vi "Scope_5782_6channel_IQ_PID_Quench.vi"() -> ()   [LabVIEW 2018]
uses:
  FPGA/DataMode.ctl
  <vilib>/Analysis/4window.llb/windowTd.ctl
  Host/Scope/controls/power_spectrum_unit.ctl
  Host/Scope5782/Scope/controls/5782_trigger_type.ctl
  Host/Scope/controls/Data_calc_mode.ctl
  Host/Scope/controls/Data_display_mode.ctl
  Host/Scope/controls/Graph_references.ctl
  Host/Scope/controls/graph_controls.ctl
  Host/Scope/controls/Channel_select_2fpga.ctl
  FPGA/PID/PID control enabled type.ctl
  <vilib>/userdefined/High Color/nirio_resource_hc.ctl
  Host/Scope/controls/All FP controls.ctl
  Host/Scope/controls/Output scale.ctl
  Host/Scope/controls/host_transfer_speed.ctl
  FPGA/cavity model/Piezo setting.ctl
  Host/Scope/controls/w12 scale.ctl
  Host/Scope/controls/FFT buffer type.ctl
  Host/Communication/Driver/RemoteConnection/RemoteReferences.ctl
  Host/FpgaRef/FpgaRef5761/ClockSource_5761.ctl
  Host/INI files/Settings file IQ PID/SettingsFileIQpid.lvclass
  C:/PXIe/InProgress/source2/Host/INI files/Settings file base/SettingsFile.lvclass
  Host/Communication/Driver/RemoteConnection/RemoteConnection.lvclass
  Host/Scope/Scope5782_six_channel/Scope5782_six_channel.lvclass
  C:/PXIe/InProgress/source2/Host/Scope/ScopeBase/ScopeBase.lvclass
  FPGA/fpga_settings.ctl
  Host/INI files/Settings file base/Save event.ctl
  Host/Scope/Scope5782_six_channel/Scope5782_six_channel.lvclass/Scope5782_six_channel.ctl
  Host/Scope/controls/ScopeMode.ctl
  Host/FpgaRef/FpgaRef5761/FpgaRef5761.lvclass
  C:/PXIe/InProgress/source2/Host/FpgaRef/FpgaRefBase/FpgaRefBase.lvclass
  Host/FpgaRef/FpgaRef5782/FpgaRef5782.lvclass
  Host/Communication/global_stop.vi
  <vilib>/FPGAPlugInAG/PXIe-7975R/niLvFpga_Open_PXIe-7975R.vi
  <vilib>/rvi/interface/common/dynamic/niFpgaDynamicAddResources.vi
  <vilib>/Utility/error.llb/Error Cluster From Error Code.vi
  <vilib>/rvi/errors/niLvFpgaAdjustHostInterfaceError.vi
  Host/Communication/response.ctl
  Host/Communication/driver_status.ctl
  <vilib>/rvi/interface/nirviOpenFPGA/nirviOpenFPGA.xnode
  FPGA Bitfiles/FPGAmain_5782_IQ_PID_PtIU9Q++q2U.lvbitx
  FPGA Bitfiles/FPGAmain_5782_IQ_PID_Quench_umIfVrlQf5Q.lvbitx
  FPGA Bitfiles/FPGAmain_5761_zuew0qNtRjU.lvbitx
  <vilib>/rvi/interface/nirviReadWriteControl/nirviReadWriteControl.xnode
  <vilib>/rvi/FXPMathLib/FxpInterpret/XNode/nifxpmath_Interpret.xnode
  Host/Communication/Driver/TcpServerDriver/TcpServerDriver.lvclass
  Host/Scope/ScopeBase/ScopeBase.lvclass
  Host/INI files/Settings file base/SettingsFile.lvclass
  NiFpgaLv.dll
  <vilib>/rvi/interface/Simulation/niFpgaSimulationCallBeginRW.vi
  Host/FpgaRef/FpgaRefBase/FpgaRefBase.lvclass
  <vilib>/Analysis/NI_AALPro.lvlib
panel:
  out "magnitude":cluster{"f0":dbl, "df":dbl, "magnitude":dbl[]}(graph)
  in  "quench":bool
  out "Lower graph":dbl[][](graph)
  out "Upper graph":dbl[][](graph)
  out "Upper chart":dbl[][](graph)
  in  "Hold plot lower":bool caption="Hold plot"
  in  "Update once lower":bool
  in  "Hold plot upper":bool caption="Hold plot"
  in  "Update once upper":bool
  in  "FFT buffer size":T1
  in  "Transfer speed":T2
  out "All FP controls":T3
  in  "Show buffers":bool
  out "Adaptive FF graph":dbl[][](graph)
  in  "Tab Control":T4(tab)
  in  "Samples before reset":u32
  in  "b":fxp<+/-,16,2>
  in  "a":fxp<+/-,16,2>
  in  "Fequency [kHz]":dbl format="%#_8g"
  in  "I Feedback":T5
  in  "Ki*T AM":fxp<+/-,32,6> caption="Ki*T"
  in  "Kd/T AM":fxp<+/-,32,11> caption="Kd/T"
  in  "Kp AM":fxp<+/-,32,6> caption="Kp"
  in  "Feedback delay":u32
  in  "Trigger delay":u32
  in  "Acquire samples":u32
  in  "Kp Q":fxp<+/-,32,6> caption="Kp"
  in  "Kd/T  Q":fxp<+/-,32,11> caption="Kd/T"
  in  "Ki*T Q":fxp<+/-,32,6> caption="Ki*T"
  in  "Q Feedback":T5
  in  "Host scale 5761":T6 caption="Host scale"
  in  "Input scale 5761":T6 caption="Input scale"
  in  "Host scale":T6
  in  "Input scale":T6
  in  "Output scale":T6
  in  "ch2 DC offset":dbl caption="DC offset\nChannel 2"
  in  "ch3 DC offset":dbl caption="DC offset\nChannel 3"
  in  "ch0 DC offset 2":dbl caption="DC offset\nChannel 0"
  in  "ch1 DC offset 2":dbl caption="DC offset\nChannel 1"
  in  "ch0 DC offset":dbl caption="DC offset\nChannel 0"
  in  "ch1 DC offset":dbl caption="DC offset\nChannel 1"
  in  "Setpoint":path
  in  "Feed forward":path
  in  "show setpoint":bool
  in  "show feedforward":bool
  in  "Setpoint enabled":bool
  in  "Piezo":T7
  in  "w0":dbl
  in  "Virtual cavity":bool
  in  "K2":dbl
  in  "Q2":dbl
  in  "w2":dbl
  in  "K3":dbl
  in  "Q3":dbl
  in  "w3":dbl
  in  "S":dbl=0.001 min=0.001 max=1000.0 format="%#_12g"
  in  "K1":dbl
  in  "Q1":dbl
  in  "w1":dbl
  in  "R1":dbl
  in  "w12":dbl format="%#_12g"
  in  "Cavity model":bool
  in  "Cal":bool
  in  "Test":bool
  in  "Q0 - D":dbl
  in  "Q0 - B":dbl
  in  "Q0 - E":dbl
  in  "Q0 - C":dbl
  in  "Q0 - A":dbl
  in  "sigm":dbl
  in  "Nforget":i32
  in  "Q0 identify":bool
  in  "Max output set":dbl min=0.0 max=16383.0
  out "Amp1":fxp<+,16,14>
  in  "Reset Quench Warning":bool
  in  "Measure Tau at Time":u32
  in  "Tau set":fxp<+/-,32,13>
  in  "Enable":bool
  out "Tau [µs]":fxp<+/-,64,26>
  out "Quench_Warning":bool
  out "Tau_set":fxp<+/-,32,13>
  in  "Input delay 5782":u32
  in  "Input delay 5761":u32
  in  "Count to skip 5782, stage 1":u32
  in  "Count to skip 5761, stage 1":u32
  in  "Count to skip 5782, stage 2":u32
  in  "Count to skip 5782, stage 3":u32
  in  "Count to skip 5761, stage 2":u32
  in  "Count to skip 5761, stage 3":u32
  in  "Vfi Vfq LP filter cut off frequency":dbl caption="MHz" min=0.0 max=10000.0
  in  "Vi Vq LP  filter cutoff fequency":dbl caption="MHz" min=0.0 max=10000.0
  in  "ch3 delay":dbl caption="ns" min=0.0 max=10000.0
  in  "ch1 delay":dbl caption="ns" min=0.0 max=10000.0
  in  "dw LP filter cut off frequency":dbl caption="MHz" min=0.0 max=10000.0
  in  "w12 LP  filter cutoff fequency":dbl caption="MHz" min=0.0 max=10000.0
  in  "dw scale":T8
  in  "w12 scale":T8
  in  "w12 - dt":dbl min=100.0 max=10000000.0
  in  "Calculate w12":bool
  in  "w12 - a":dbl format="%#_12g"
  in  "w12 - b":dbl
  in  "5761 resource":T9="PXI2Slot11"
  in  "5782 resource":T9="PXI2Slot18"
  in  "Output enabled":bool=TRUE
  in  "Output delay delta":dbl(slide) scale=0.0..6.0
  in  "Output delay":dbl(slide) scale=0.0..6.0
  in  "Output mixer fequency [MHz]":dbl
  in  "Trigger":T10
  in  "Mode":T11
  in  "Mixer freq [MHz]":dbl
  in  "Unwrap phase":bool
  in  "#bins":i32=1 min=1 max=16
  in  "Unit":T12
  in  "Window":T13=1 items=["Rectangle"=0, "Hanning"=1, "Hamming"=2, "Blackman-Harris"=3, "Exact Blackman"=4, "Blackman"=5, "Flat Top"=6, "4 Term B-Harris "=7, "7 Term B-Harris"=8, "Low Sidelobe"=9, "Blackman Nuttall"=11, "Triangle"=30, "Bartlett-Hanning"=31, "Bohman"=32, "Parzen"=33, "Welch"=34, "Kaiser"=60, "Dolph-Chebyshev"=61, "Gaussian"=62]
  in  "Chart length":i32=400000
  in  "Trigmode":enum32{"Triggered", "Continuous"}(radio)
  in  "Reference for phase":T14
  in  "Graph_refs":T15
  out "Lower chart":dbl[][](graph)
  in  "Buffer":T17
  in  "Display":T18
  out "stop 2":bool
  in  "Zoom freq X":bool
  in  "Zoom freq Y":bool
  in  "Zoom time Y":bool
  in  "Zoom time X":bool
  in  "Samples per 5782 record":i32
  in  "Phase offset (deg)":dbl
  in  "Fequency [MHz]":dbl format="%#_8g"
  out "freqdata":cluster{"f0":dbl, "df":dbl, "magnitude":dbl[]}[](graph)
  in  "Rumode":bool
  in  "Singleshot":bool
  out "error IO":errorcluster
  in  "stop":bool
  # "FPGA setup"
  # "ns"
  # "Output delay"
  # "Auto Zoom"
  # "FFT"
  # "Auto Zoom"
  # "Amplitude modulation"
  # "5785"
  # "5761"
  # "5782"
  # "V"
  # "V"
  # "5761"
  # "V"
  # "V"
  # "V"
  # "V"
  # "Simulated data"
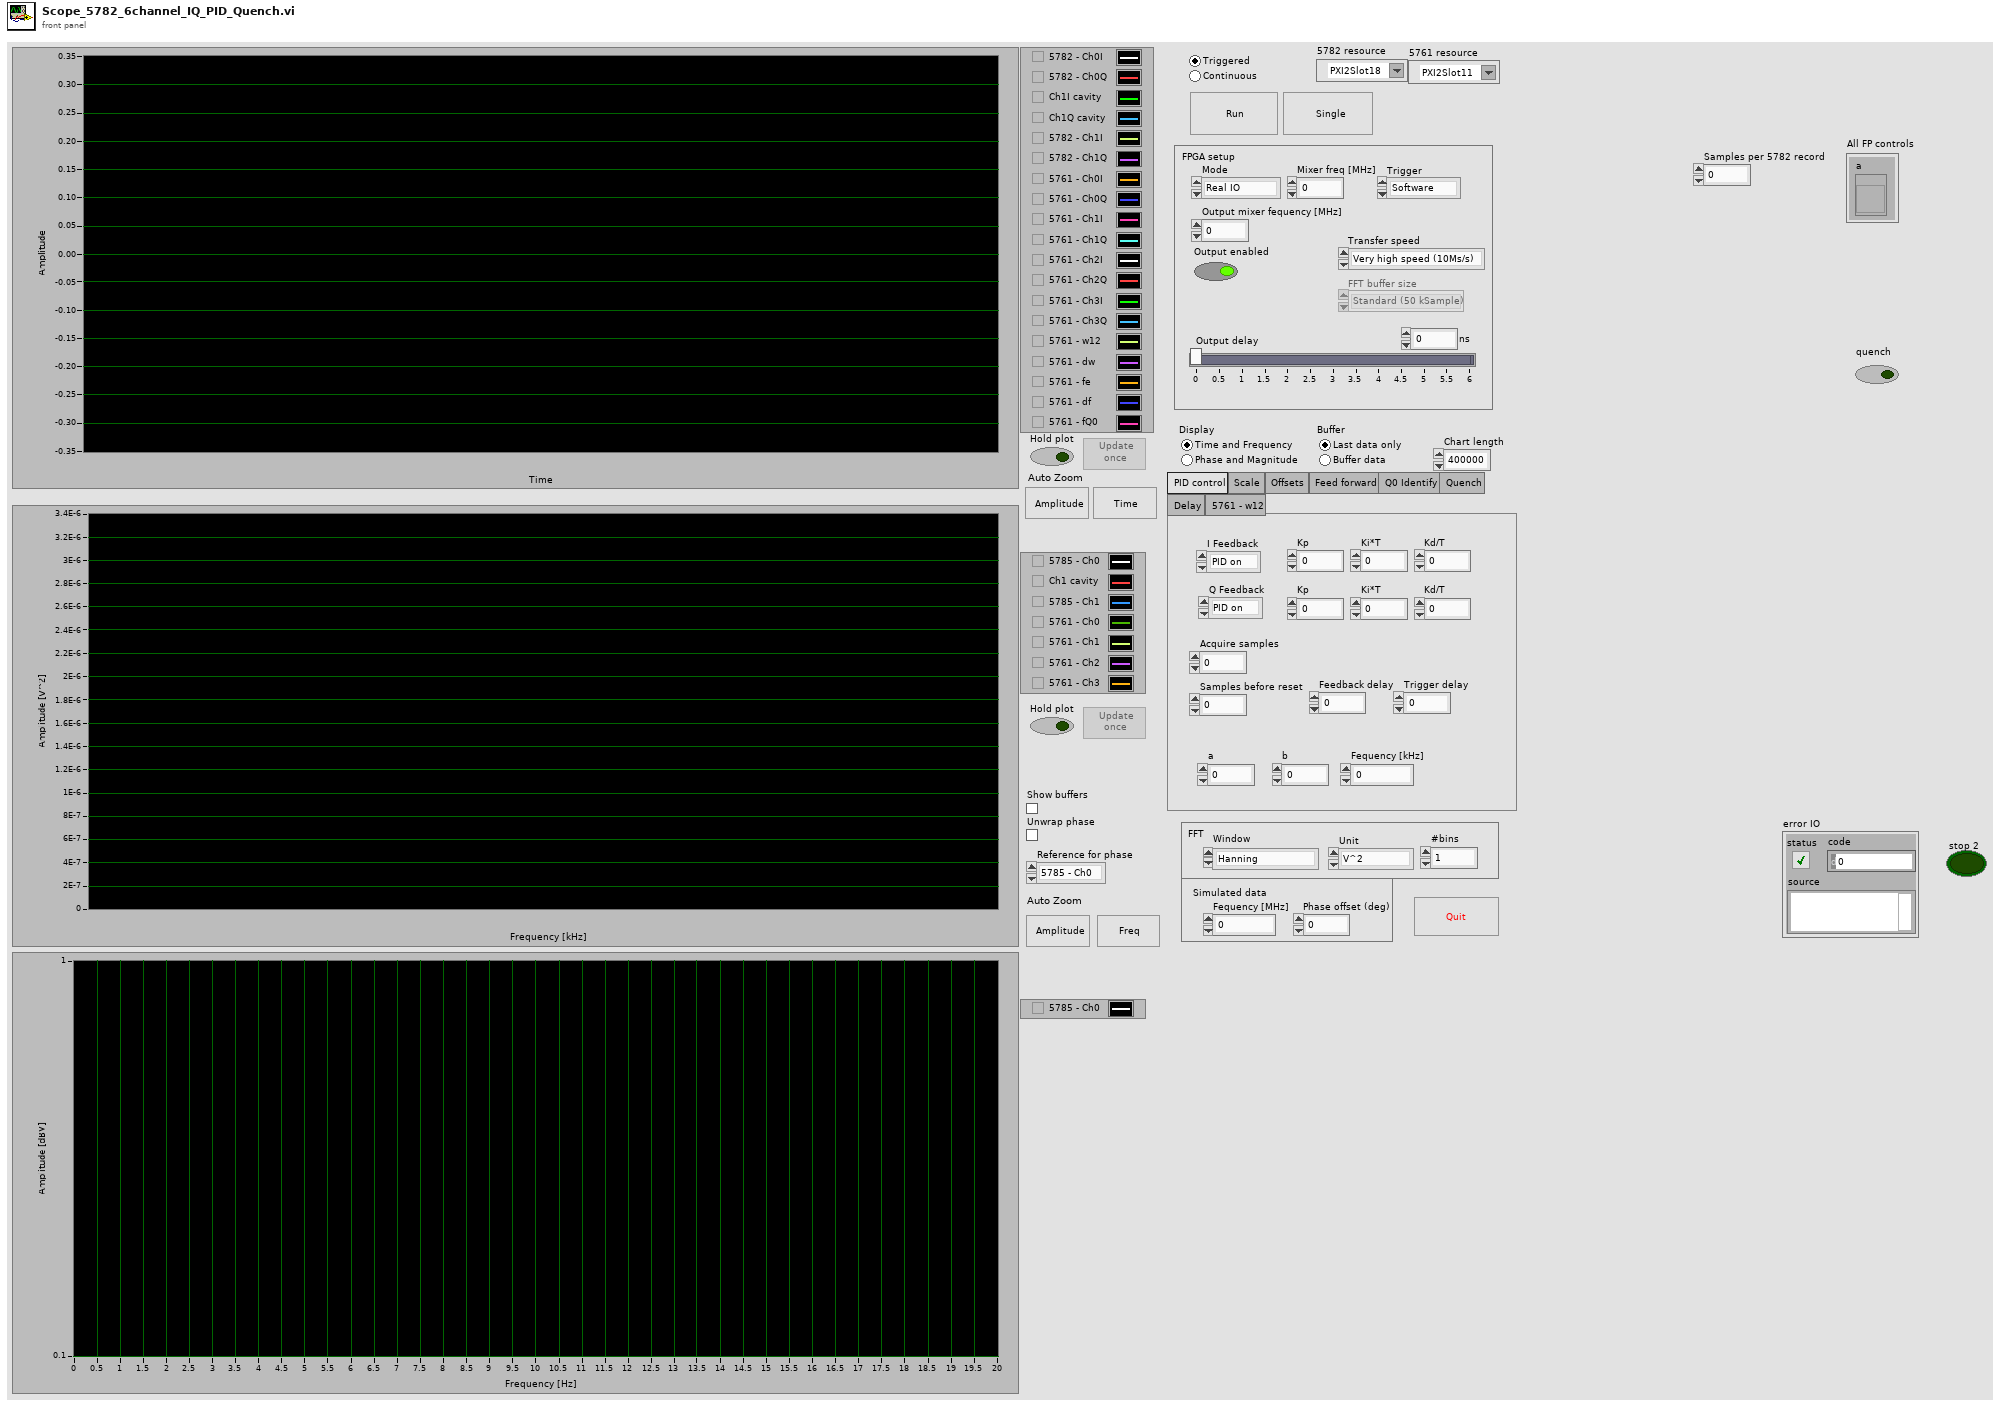
[diagram p1: front panel]
types:
  T1 = typedef "FFT buffer type.ctl" = enum16{"Standard (50 kSample)", "Long (250 kSample)"}
  T2 = typedef "host_transfer_speed.ctl" = enum16{"Very high speed (10Ms/s)", "High speed (1Ms/s)", "Low speed (50kS/s)", "Ultra low speed (20kS/s)"}
  T3 = typedef "All FP controls.ctl" = cluster{"ch1 DC offset":refnum<vi>, "ch0 DC offset":refnum<vi>, "ch1 DC offset 2":refnum<vi>, "ch0 DC offset 2":refnum<vi>, "ch3 DC offset":refnum<vi>, "ch2 DC offset":refnum<vi>, "Feedback Q":refnum<vi>, "Ki*T Q":refnum<vi>, "Kd/T  Q":refnum<vi>, "Kp Q":refnum<vi>, "Acquire samples":refnum<vi>, "Trigger delay":refnum<vi>, "Feedback delay":refnum<vi>, "Kp AM":refnum<vi>, "Kd/T AM":refnum<vi>, "Ki*T AM":refnum<vi>, "Feedback I":refnum<vi>, "#bins":refnum<vi>, "Window":refnum<vi>, "Unit":refnum<vi>, "Input delay 5761":refnum<vi>, "Input delay 5785":refnum<vi>, "S":refnum<vi>, "K1":refnum<vi>, "Q1":refnum<vi>, "R1":refnum<vi>, "w12":refnum<vi>, "Cavity model":refnum<vi>, "w1":refnum<vi>, "Mode":refnum<vi>, "Trigger":refnum<vi>, "Output mixer fequency [MHz]":refnum<vi>, "Output delay":refnum<vi>, "Mixer freq [MHz]":refnum<vi>, "Triggered":refnum<vi>, "Continuous":refnum<vi>, "Output scale":refnum<vi>, "Host scale":refnum<vi>, "Input scale":refnum<vi>, "IIR filter cutoff fequency [MHz]":refnum<vi>, "Host scale 5761":refnum<vi>, "Virtual cavity":refnum<vi>, "Input scale 5761":refnum<vi>, "Tranfer speed":refnum<vi>, "Count to skip 5782, stage 1":refnum<vi>, "Count to skip 5761, stage 1":refnum<vi>, "K2":refnum<vi>, "w2":refnum<vi>, "K3":refnum<vi>, "Q3":refnum<vi>, "Q2":refnum<vi>, "w3":refnum<vi>, "w0":refnum<vi>, "Piezo":refnum<vi>, "Measure Tau at Time":refnum<vi>, "Tau set":refnum<vi>, "Count to skip 5761, stage 2":refnum<vi>, "Count to skip 5761, stage 3":refnum<vi>, "Count to skip 5782, stage 2":refnum<vi>, "Count to skip 5782, stage 3":refnum<vi>, "Fequency [kHz]":refnum<vi>, "a":refnum<vi>, "b":refnum<vi>, "w12 - b":refnum<vi>, "w12 - a":refnum<vi>, "w12 - dt":refnum<vi>, "w12 scale":refnum<vi>, "dw scale":refnum<vi>, "w12 LP  filter cutoff fequency":refnum<vi>, "dw LP filter cut off frequency":refnum<vi>, "ch1 delay":refnum<vi>, "ch3 delay":refnum<vi>, "Vi Vq LP  filter cutoff fequency":refnum<vi>, "Vfi Vfq LP filter cut off frequency":refnum<vi>, "Q0 - C":refnum<vi>, "sigm":refnum<vi>, "Q0 - A":refnum<vi>, "Q0 - E":refnum<vi>, "Nforget":refnum<vi>, "Q0 - B":refnum<vi>, "Q0 - D":refnum<vi>, "Samples before reset":refnum<vi>}
  T4 = enum32{"PID control", "Scale", "Offsets", "Feed forward", "Cavity model", "Q0 Identify", "Quench", "Delay", "5761 - w12"}
  T5 = typedef "PID control enabled type.ctl" = enum16{"PID on", "Ref", "Zero"}
  T6 = typedef "Output scale.ctl" = enum16{"x1", "x2", "x4", "x8", "x16", "x32"}
  T7 = typedef "Piezo setting.ctl" = enum16{"Off", "On - Ch 0", "On - Ch 1"}
  T8 = typedef "w12 scale.ctl" = enum16{"x1", "1/2", "1/4", "1/8", "1/16", "1/32", "1/64", "1/128", "1/256", "1/512", "1/1024", "1/2048", "1/4096", "1/8192"}
  T9 = typedef "nirio_resource_hc.ctl" = tag
  T10 = typedef "5782_trigger_type.ctl" = enum16{"Software", "Trigger input"}
  T11 = typedef "DataMode.ctl" = enum16{"Real IO", "Simulated"}
  T12 = typedef "power_spectrum_unit.ctl" = enum16{"V^2", "V", "dBV"}
  T13 = typedef "NI_AALPro.lvlib/windowTd.ctl" = u32
  T14 = typedef "Channel_select_2fpga.ctl" = enum16{"5785 - Ch0", "5785 - Ch1 cavity", "5785 - Ch1", "5761 - Ch0", "5761 - Ch1", "5761 - Ch2", "5761 - Ch3"}
  T15 = typedef "Graph_references.ctl" = cluster{"upper":T16, "lower":T16, "Freq graph":refnum<vi>, "Adaptive FF graph":refnum<vi>}
  T16 = typedef "graph_controls.ctl" = cluster{"Graph":refnum<vi>, "Time btn":refnum<vi>, "Amplitude btn":refnum<vi>, "Chart":refnum<vi>}
  T17 = typedef "Data_display_mode.ctl" = enum32{"Last data only", "Buffer data"}
  T18 = typedef "Data_calc_mode.ctl" = enum32{"Time and Frequency", "Phase and Magnitude"}
  T19 = typedef "ClockSource_5761.ctl" = enum8{"Internal Clock PLL Off", "Internal Clock PLL On (CLK_IN)", "External Clock (CLK_IN)", "Internal Clock PLL On (IoModSyncClk)", "External Clock (IoModSyncClk)"}
  T20 = typedef "RemoteConnection.lvclass/RemoteReferences.ctl" = cluster{"a":refnum<vi>, "b":refnum<vi>, "fm":refnum<vi>, "Output delay":refnum<vi>, "Output delay delta":refnum<vi>}
  T21 = typedef "response.ctl" = cluster{"driver status":T22, "Sender":string, "Type":i32, "Variant":variant}
  T22 = typedef "driver_status.ctl" = enum16{"Normal", "Startup", "Connection lost", "Reconnected", "Timeout", "Idle", "Busy"}
  T23 = typedef "message_queue.ctl" = refnum<queue>
  T24 = enum8{"Internal Clock PLL Off", "Internal Clock PLL On (REF IN)", "External Clock (CLK_IN)", "Internal Clock PLL On (IoModSyncClk)"}
  T25 = typedef "INI Save Event.ctl" = refnum<user-event>
  T26 = typedef "Save event.ctl" = cluster{"Automatic":bool, "Save":bool}
  T27 = typedef "fpga_settings.ctl" = enum16{"Feedback Enable", "New FIR coeffs", "FIR shift", "Enable filter", "Set Downsample", "Downsample", "CIC Gain", "Record length", "Trigger samples", "Quiet time", "a_am", "b_am", "Use fixed delay", "fixed sin_fi", "fixed cos_fi", "Ki*Tau", "Kp", "Kd_Tau", "Fi_start", "Fi_delta", "DC_offs 0", "DC_offs 1", "DC_offs 2", "DC_offs 3", "Ki*Tau am", "Kp am", "Kd_Tau am", "Feedback AM", "Trigger delay", "Feedback delay", "Setpoint enable", "Beam enable", "Samples to acquire", "Cavity Enable", "Cavity C1", "Cavity C2", "Cavity C3", "Cavity C4", "Cavity C5", "Input delay", "Ki*Tau Q", "Kp Q", "Kd_Tau Q", "Adaptive FF enable", "Feedforward a0", "Feedforward b0", "FF src adress", "FF dest adress", "Output scale", "Input scale", "Host scale", "FF_IIR b0", "FF_IIR b1", "FF_IIR b2", "FF_IIR-a1", "FF_IIR-a2", "Enable HW trigger", "Virtual cavity", "Samples to skip", "Samples to skip 2", "Samples to skip 3", "Cavity C3_2", "Cavity C4_2", "Cavity C5_2", "Cavity C3_3", "Cavity C4_3", "Cavity C5_3", "Cavity_w0_dt", "Piezo setting", "Quench t0", "Quench tau set", "Quench enabled", "Quench reset", "PID enabled I", "PID enabled Q", "Cavity filter a", "Cavity filter b", "Disable e(n)", "FF e(n) src address", "FF first address", "FF last address", "FF PID first address", "FF PID last address", "Amp IIR b0", "Amp IIR b1", "Amp IIR b2", "Amp IIR-a1", "Amp IIR-a2", "Adaptation factor", "Inv Amp LP b0", "Inv Amp LP b1", "Inv Amp LP b2", "Inv Amp LP-a1", "Inv Amp LP-a2", "Inv Amp c0", "Inv Amp c1", "Inv Amp c2", "Inv Amp c3", "Inv Amp c4", "Inv Amp -d1", "Inv Amp -d2", "Inv Amp -d3", "Inv Amp -d4", "w12_a", "w12_b", "w12_dt", "w12_scale", "dw_scale", "Extra output select", "Extra fi sin", "Extra fi cos", "Extra output scale", "Quench max output", "Samples before reset"}
  T28 = enum8{"Enabled", "Disabled", "Disabled and Grayed Out"}
  T29 = typedef "ScopeMode.ctl" = enum16{"Stopped", "Single", "Running", "Continuous"}
  T30 = typedef "PlotUpdate type.ctl" = enum16{"None", "Graph", "Chart", "Freq"}
  T31 = typedef "Feedforward.ctl" = cluster{"Beam I":dbl[], "Beam Q":dbl[], "Feedforward I":dbl[], "Feedforward Q":dbl[], "Setpoint I":dbl[], "Setpoint Q":dbl[]}
  T32 = typedef "Scope5782_six_channel.lvclass/Q0 params.ctl" = cluster{"Nforget":i32, "sigm":dbl, "Q0 - A":dbl, "Q0 - B":dbl, "Q0 - C":dbl, "Q0 - D":dbl, "Q0 - E":dbl, "Test":bool, "Cal":bool}
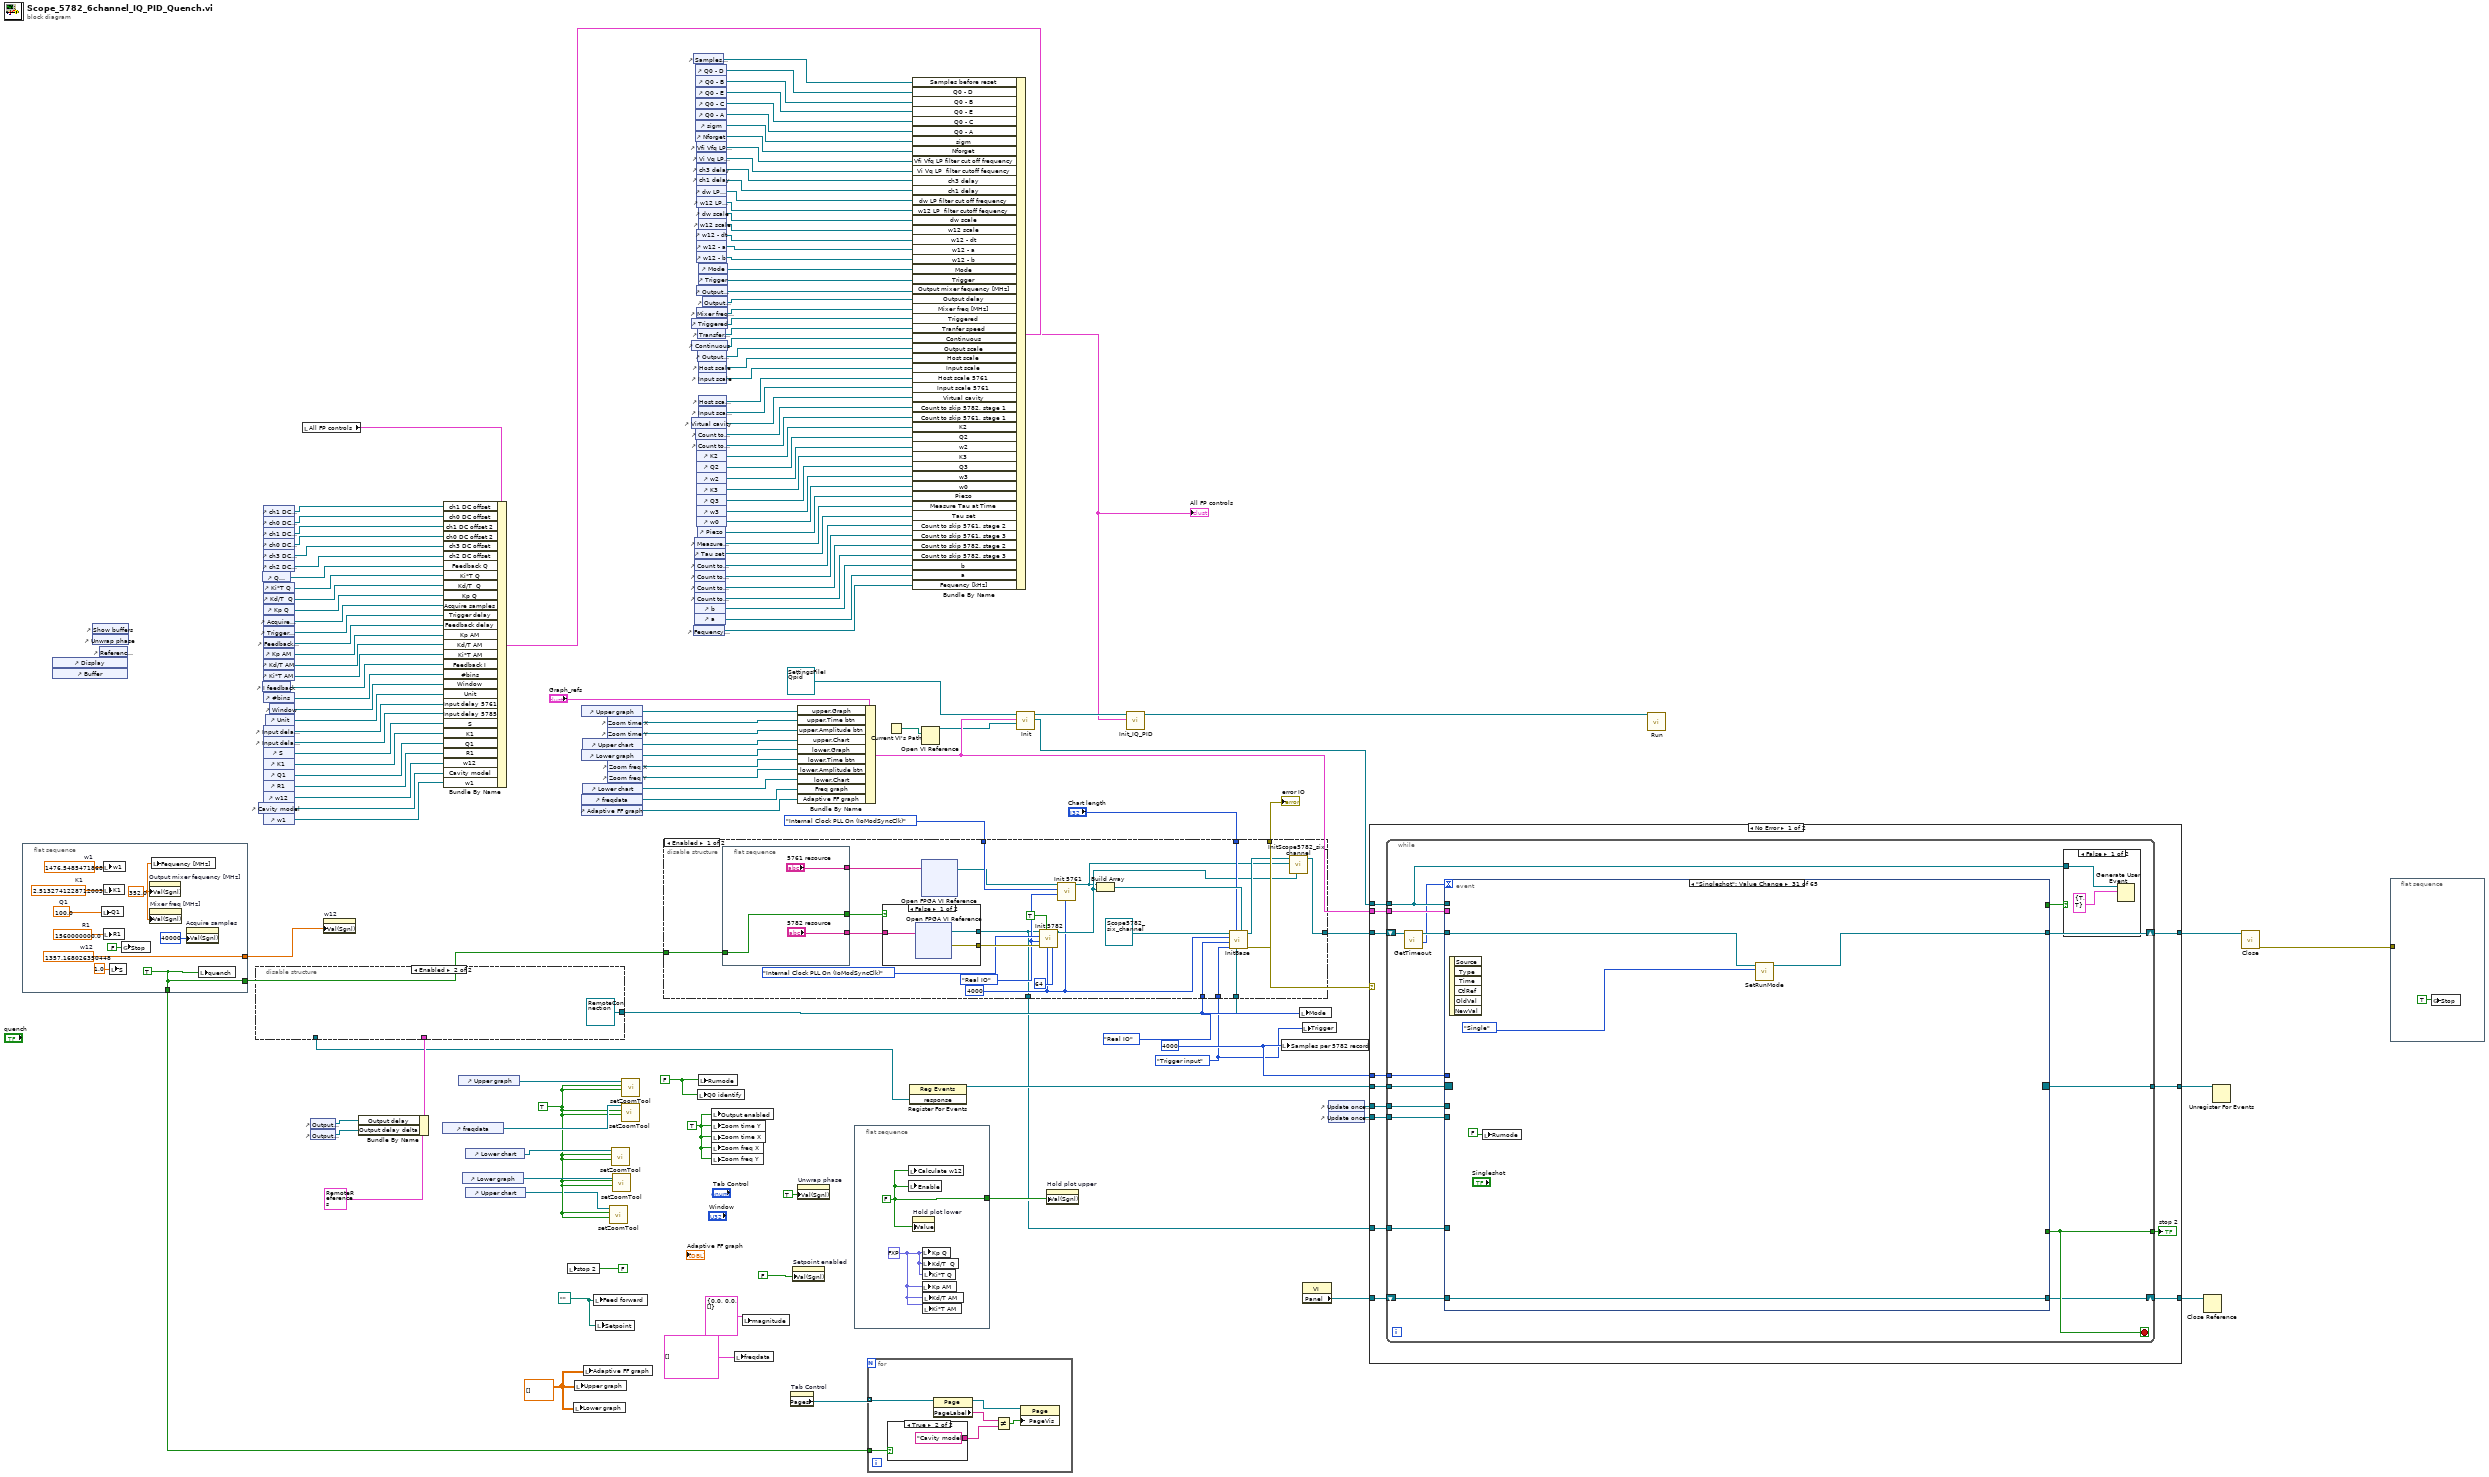
[diagram p0: block diagram]
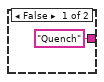
[diagram p2: hidden frame]
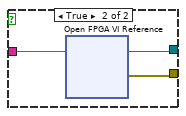
[diagram p3: hidden frame]
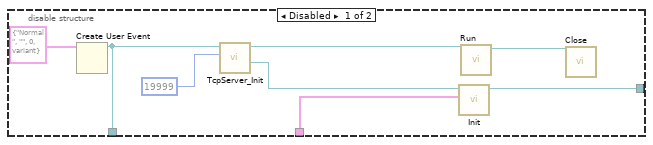
[diagram p5: hidden frame]
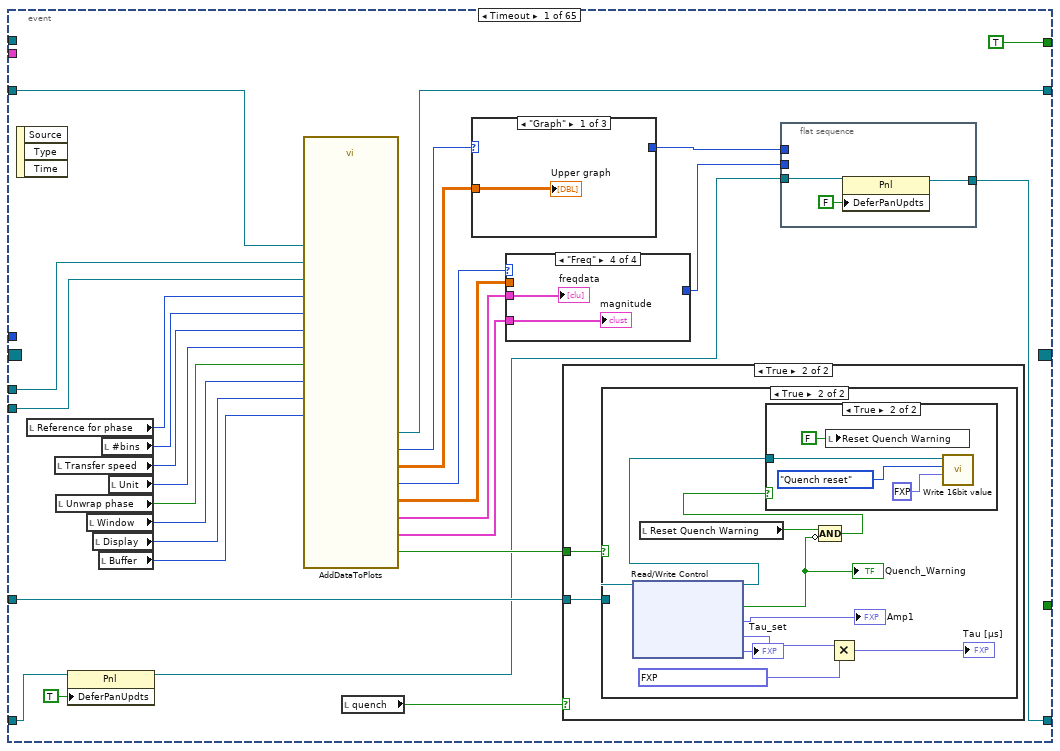
[diagram p7: hidden frame]
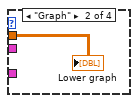
[diagram p12: hidden frame]
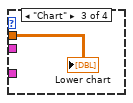
[diagram p13: hidden frame]
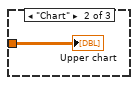
[diagram p14: hidden frame]
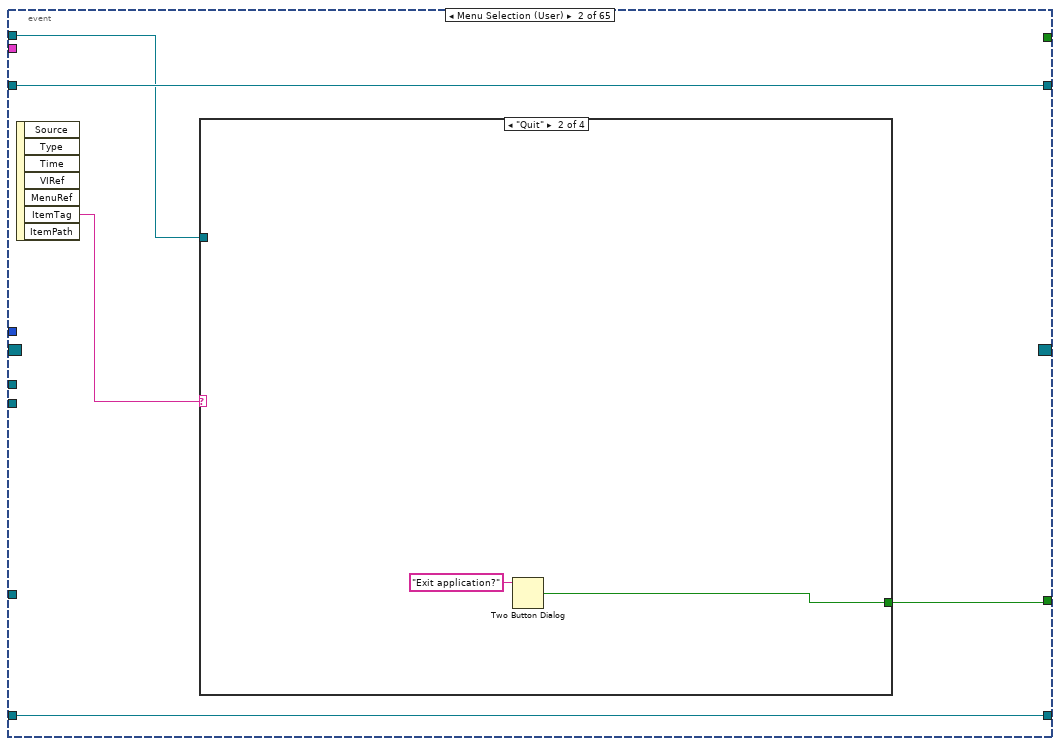
[diagram p16: hidden frame]
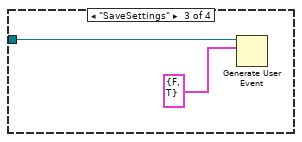
[diagram p18: hidden frame]
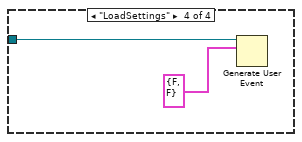
[diagram p19: hidden frame]
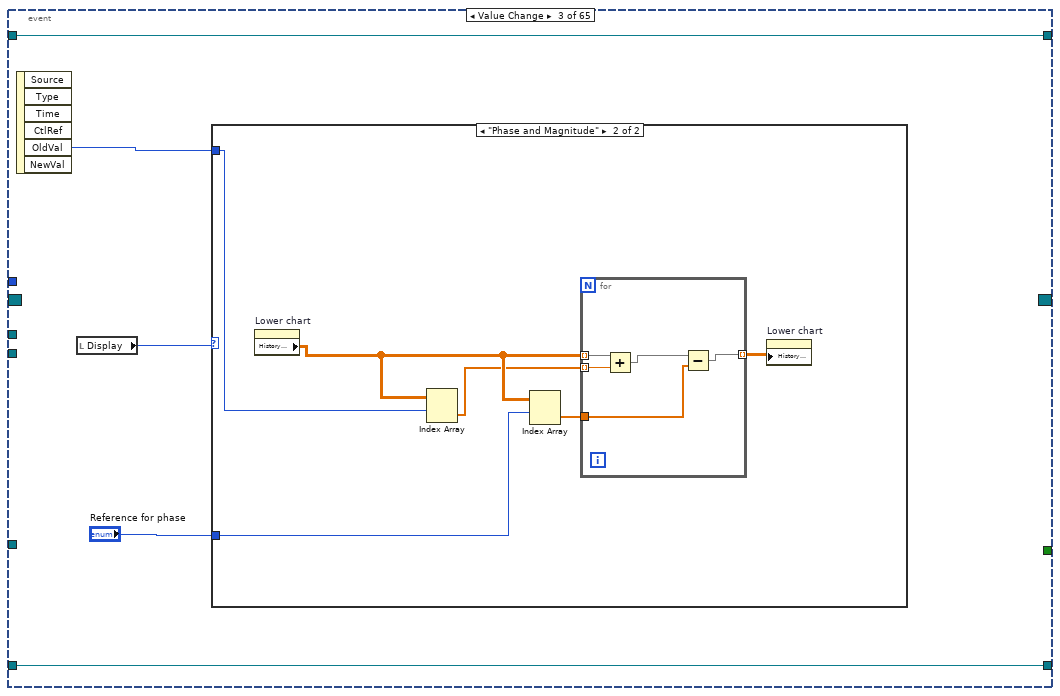
[diagram p20: hidden frame]
diagram:
  w117 = DataMode."Real IO" ("Mode")
  w119 = path "" ("Feed forward")
  w116 = 5782_trigger_type."Trigger input" ("Trigger")
  w30 = TRUE ("Zoom  X")
  w122 = TRUE ("Rumode")
  w121 = 4000 ("Samples to aqcuire")
  w32 = dbl[][] [] ("Timedata")
  w3 = FALSE ("Rumode")
  n1 = flat-sequence {
    tunnel: [w149] -> w64
    tunnel: [w146] -> w25
    tunnel: [w146] -> w24
    frame #0 {
      w146 = TRUE ("quench")
      w147 = 352.0 ("Value (Signaling)")
      w151 = 2.5132741228712003  # K1
      w150 = 100.0  # Q1
      w152 = 1476.54854718683  # w1
      w153 = 1560000000.0  # R1
      w149 = 1357.168026350448  # w12
      n2 = local write "Q1"(w150) -> ()
      n3 = local write "w1"(w152) -> ()
      n4 = local write "K1"(w151) -> ()
      n5 = local write "R1"(w153) -> ()
      n6 = local write "S"(1.0 ("S")) -> ()
      n7 = global write "global_stop.vi" "Stop"(FALSE ("Stop")) -> ()
      n8 = property on="Output mixer fequency [MHz]" class="DigNum (strict)"("Val(Sgnl)"=w147) -> ()  [unwired: 2 in, 2 out]
      n9 = property on="Mixer freq [MHz]" class="DigNum (strict)"("Val(Sgnl)"=w147) -> ()  [unwired: 2 in, 2 out]
      n10 = local write "Fequency [MHz]"(w147) -> ()
      n11 = property on="Acquire samples" class="DigNum (strict)"("Val(Sgnl)"=u32 40000 ("Value (Signaling)")) -> ()  [unwired: 2 in, 2 out]
      n12 = local write "quench"(w146) -> ()
    }
  }
  n13 = control-ref of="Display"() -> ()  [unwired: 1 out]
  n14 = control-ref of="Buffer"() -> ()  [unwired: 1 out]
  n15 = control-ref of="Show buffers"() -> ()  [unwired: 1 out]
  n16 = control-ref of="Unwrap phase"() -> ()  [unwired: 1 out]
  n17 = control-ref of="Reference for phase"() -> ()  [unwired: 1 out]
  n18 = control-ref of="Cavity model"() -> (w81:refnum<vi>)
  n19 = control-ref of="Q Feedback"() -> (w102:refnum<vi>)
  n20 = control-ref of="I feedback"() -> (w92:refnum<vi>)
  n21 = control-ref of="Ki*T Q"() -> (w101:refnum<vi>)
  n22 = control-ref of="Kd/T  Q"() -> (w100:refnum<vi>)
  n23 = control-ref of="Kp Q"() -> (w99:refnum<vi>)
  n24 = control-ref of="Acquire samples"() -> (w98:refnum<vi>)
  n25 = control-ref of="Trigger delay"() -> (w97:refnum<vi>)
  n26 = control-ref of="Feedback delay"() -> (w96:refnum<vi>)
  n27 = control-ref of="Kp AM"() -> (w95:refnum<vi>)
  n28 = control-ref of="Kd/T AM"() -> (w94:refnum<vi>)
  n29 = control-ref of="Ki*T AM"() -> (w93:refnum<vi>)
  n30 = control-ref of="#bins"() -> (w91:refnum<vi>)
  n31 = control-ref of="Input delay 5761"() -> (w88:refnum<vi>)
  n32 = control-ref of="Input delay 5782"() -> (w87:refnum<vi>)
  n33 = control-ref of="S"() -> (w86:refnum<vi>)
  n34 = control-ref of="K1"() -> (w85:refnum<vi>)
  n35 = control-ref of="Q1"() -> (w84:refnum<vi>)
  n36 = control-ref of="R1"() -> (w83:refnum<vi>)
  n37 = control-ref of="w12"() -> (w82:refnum<vi>)
  n38 = control-ref of="w1"() -> (w80:refnum<vi>)
  n39 = control-ref of="ch1 DC offset"() -> (w108:refnum<vi>)
  n40 = control-ref of="ch0 DC offset"() -> (w107:refnum<vi>)
  n41 = control-ref of="ch1 DC offset 2"() -> (w106:refnum<vi>)
  n42 = control-ref of="ch0 DC offset 2"() -> (w105:refnum<vi>)
  n43 = control-ref of="ch3 DC offset"() -> (w104:refnum<vi>)
  n44 = control-ref of="ch2 DC offset"() -> (w103:refnum<vi>)
  n45 = control-ref of="Unit"() -> (w89:refnum<vi>)
  n46 = control-ref of="Window"() -> (w90:refnum<vi>)
  n47 = local read "All FP controls"() -> (w109:T3)
  n48 = control-ref of="Output delay"() -> (w125:refnum<vi>)
  n49 = control-ref of="Output delay delta"() -> (w124:refnum<vi>)
  n50 = property on="w12" class="DigNum (strict)"("Val(Sgnl)"=w64) -> ()  [unwired: 2 in, 2 out]
  n51 = Bundle By Name(cluster=T20 {"a"=refnum, "b"=refnum, "fm"=refnum, "Output delay"=refnum, "Output delay delta"=refnum} ("refs"), "Output delay"=w125, "Output delay delta"=w124) -> (w129:T20)
  n52 = disable-structure shown="Enabled" {
    disable-tunnel: w129 -> [w162 _]
    disable-tunnel: [w157 _] -> w127
    disable-tunnel: [w155 refnum<class "RemoteConnection.lvclass"> refnum ("RemoteConnection")] -> w115
    frame Disabled {
      n53 = Create User Event(user event datatype=T21 {"driver status"=enum."Normal", "Sender"="", "Type"=0, "Variant"=variant} ("response")) -> (user event=w157:refnum<user-event>)  [unwired: 1 in, 1 out]
      n54 = call "TcpServer_Init.vi"("local port"=u16 19999, "response event"=w157) -> ("Message queue"=w161:T23, "TcpServerDriver"=w159:refnum<class "TcpServerDriver.lvclass">)  [unwired: 8 in]
      n55 = call "Init.vi"("refs"=w162, "server queue"=w161) -> ("RemoteConnection"=w155:refnum<class "RemoteConnection.lvclass">)  [unwired: 9 in]
      n56 = call-dynamic "Run.vi"("BaseDriver in"=w159) -> ("BaseDriver out"=w160:refnum<class "TcpServerDriver.lvclass">)  [unwired: 9 in, 1 out]
      n57 = call-dynamic "Close.vi"("BaseDriver in"=w160) -> ()  [unwired: 9 in, 2 out]
    }
    frame Enabled {
    }
  }
  n58 = control-ref of="freqdata"() -> (w140:refnum<vi>)
  n59 = Bundle By Name(cluster=w109, "ch1 DC offset"=w108, "ch0 DC offset"=w107, "ch1 DC offset 2"=w106, "ch0 DC offset 2"=w105, "ch3 DC offset"=w104, "ch2 DC offset"=w103, "Feedback Q"=w102, "Ki*T Q"=w101, "Kd/T  Q"=w100, "Kp Q"=w99, "Acquire samples"=w98, "Trigger delay"=w97, "Feedback delay"=w96, "Kp AM"=w95, "Kd/T AM"=w94, "Ki*T AM"=w93, "Feedback I"=w92, "#bins"=w91, "Window"=w90, "Unit"=w89, "Input delay 5761"=w88, "Input delay 5785"=w87, "S"=w86, "K1"=w85, "Q1"=w84, "R1"=w83, "w12"=w82, "Cavity model"=w81, "w1"=w80) -> (w79:T3)
  n60 = control-ref of="Upper graph"() -> (w141:refnum<vi>)
  n61 = control-ref of="Lower graph"() -> (w31:refnum<vi>)
  n62 = control-ref of="Lower chart"() -> (w126:refnum<vi>)
  n63 = control-ref of="Upper chart"() -> (w29:refnum<vi>)
  n64 = local write "stop 2"(FALSE ("stop 2")) -> ()
  n65 = local write "Lower graph"(w32) -> ()
  n66 = local write "Upper graph"(w32) -> ()
  n67 = control-ref of="Upper graph"() -> (w138:refnum<vi>)
  n68 = control-ref of="Lower graph"() -> (w134:refnum<vi>)
  n69 = control-ref of="freqdata"() -> (w130:refnum<vi>)
  n70 = control-ref of="Adaptive FF graph"() -> (w110:refnum<vi>)
  n71 = control-ref of="Upper chart"() -> (w135:refnum<vi>)
  n72 = control-ref of="Lower chart"() -> (w131:refnum<vi>)
  n73 = local write "Adaptive FF graph"(w32) -> ()
  n74 = local write "Feed forward"(w119) -> ()
  n75 = local write "Setpoint"(w119) -> ()
  n76 = control-ref of="Zoom time X"() -> (w137:refnum<vi>)
  n77 = control-ref of="Zoom time Y"() -> (w136:refnum<vi>)
  n78 = control-ref of="Zoom freq X"() -> (w133:refnum<vi>)
  n79 = control-ref of="Zoom freq Y"() -> (w132:refnum<vi>)
  n80 = call "setZoomTool.vi"("Zoom Y"=w30, "Zoom  X"=w30, "reference"=w29) -> ()  [unwired: 9 in]
  n81 = call "setZoomTool.vi"("Zoom Y"=w30, "Zoom  X"=w30, "reference"=w126) -> ()  [unwired: 9 in]
  n82 = call "setZoomTool.vi"("Zoom Y"=w30, "Zoom  X"=w30, "reference"=w31) -> ()  [unwired: 9 in]
  n83 = call "setZoomTool.vi"("Zoom Y"=w30, "Zoom  X"=w30, "reference"=w140) -> ()  [unwired: 9 in]
  n84 = call "setZoomTool.vi"("Zoom Y"=w30, "Zoom  X"=w30, "reference"=w141) -> ()  [unwired: 9 in]
  n85 = disable-structure shown="Enabled" {
    disable-tunnel: ClockSource_5761."Internal Clock PLL On (IoModSyncClk)" ("Clock Source") -> [w187 _]
    disable-tunnel: w117 -> [w183 _]
    disable-tunnel: w116 -> [w182 _]
    disable-tunnel: w115 -> [w181 _]
    disable-tunnel: "Chart length" -> [w180 _]
    disable-tunnel: [w179 _] -> w62
    disable-tunnel: [w175 _] -> w111
    disable-tunnel: [w164 _] -> w42
    disable-tunnel: w24 -> [w166 _]
    frame Enabled {
      w168 = u16 4000 ("Samples to aqcuire")
      w171 = DataMode."Real IO" ("Mode")
      n86 = flat-sequence {
        tunnel: ["5761 resource"] -> w185
        tunnel: ["5782 resource"] -> w184
        tunnel: [w194] -> w167
        tunnel: w166 -> [w194]
        frame #0 {
        }
      }
      n87 = case shown="False" w167 {
        tunnel: w184 -> [w190 w193]
        tunnel: [w189 w192] -> w177
        tunnel: [w188 w191] -> w164
        frame False {
          n88 = xnode "Open FPGA VI Reference"("resource name"=w190) -> ("FPGA VI Reference Out"=w188:refnum<k20>, "error out"=w189:errorcluster)  [unwired: 1 in]
        }
        frame True {
          n89 = xnode "Open FPGA VI Reference"("resource name"=w193) -> ("FPGA VI Reference Out"=w191:refnum<k20>, "error out"=w192:errorcluster)  [unwired: 1 in]
        }
      }
      n90 = xnode "Open FPGA VI Reference"("resource name"=w185) -> ("FPGA VI Reference Out"=w165:refnum<k20>)  [unwired: 1 in, 1 out]
      n91 = call "Init 5782.vi"("User Data 1"=u8 64, "Record length"=w168, "Use 1Mhz clock"=TRUE, "error in (no error)"=w177, "Mode"=w171, "Clock Source"=T24."Internal Clock PLL On (IoModSyncClk)", "FPGA ref"=w164) -> ("FpgaRef5782 Out"=w174:refnum<class "FpgaRef5782.lvclass">)  [unwired: 3 in, 1 out]
      n92 = call "Init 5761.vi"("Record length"=w168, "Mode"=w171, "Clock Source"=w187, "FPGA ref"=w165) -> ("FpgaRef5761 out"=w173:refnum<class "FpgaRef5761.lvclass">)  [unwired: 6 in, 1 out]
      n93 = Build Array(w173, w174) -> (w186:refnum<class "FpgaRefBase.lvclass">[])
      n94 = call "InitBase.vi"("FPGA refs"=w186, "RemoteConnection"=w181, "Chart length"=w180, "Trigger"=w182, "data mode"=w183, "Samples Per Trigger"=w168, "ScopeBase in"=refnum<class "Scope5782_six_channel.lvclass"> refnum ("Scope5761")) -> ("error out"=w179:errorcluster, "ScopeBase out"=w176:refnum<class "Scope5782_six_channel.lvclass">)  [unwired: 3 in]
      n95 = call "InitScope5782_six_channel.vi"("FpgaRef5782"=w174, "FpgaRef5761"=w173, "Scope5785_six_channel"=w176) -> ("Scope5785_six_channel out"=w175:refnum<class "Scope5782_six_channel.lvclass">)  [unwired: 7 in, 1 out]
    }
    frame Disabled {
    }
  }
  "error IO" <- w62
  n96 = control-ref of="Virtual cavity"() -> (w57:refnum<vi>)
  n97 = control-ref of="Triggered"() -> (w73:refnum<vi>)
  n98 = control-ref of="Continuous"() -> (w72:refnum<vi>)
  n99 = control-ref of="Samples before reset"() -> (w4:refnum<vi>)
  n100 = control-ref of="Fequency [kHz]"() -> (w26:refnum<vi>)
  n101 = control-ref of="a"() -> (w27:refnum<vi>)
  n102 = control-ref of="Measure Tau at Time"() -> (w40:refnum<vi>)
  n103 = control-ref of="Tau set"() -> (w39:refnum<vi>)
  n104 = control-ref of="Count to skip 5761, stage 2"() -> (w38:refnum<vi>)
  n105 = control-ref of="Count to skip 5761, stage 3"() -> (w37:refnum<vi>)
  n106 = control-ref of="Count to skip 5782, stage 2"() -> (w36:refnum<vi>)
  n107 = control-ref of="Count to skip 5782, stage 3"() -> (w35:refnum<vi>)
  n108 = control-ref of="b"() -> (w28:refnum<vi>)
  n109 = control-ref of="Q0 - D"() -> (w5:refnum<vi>)
  n110 = control-ref of="Q0 - B"() -> (w6:refnum<vi>)
  n111 = control-ref of="Q0 - E"() -> (w7:refnum<vi>)
  n112 = control-ref of="Q0 - C"() -> (w8:refnum<vi>)
  n113 = control-ref of="Q0 - A"() -> (w9:refnum<vi>)
  n114 = control-ref of="sigm"() -> (w10:refnum<vi>)
  n115 = control-ref of="Nforget"() -> (w11:refnum<vi>)
  n116 = control-ref of="Count to skip 5782, stage 1"() -> (w53:refnum<vi>)
  n117 = control-ref of="Vfi Vfq LP filter cut off frequency"() -> (w12:refnum<vi>)
  n118 = control-ref of="Vi Vq LP  filter cutoff fequency"() -> (w13:refnum<vi>)
  n119 = control-ref of="ch3 delay"() -> (w14:refnum<vi>)
  n120 = control-ref of="ch1 delay"() -> (w15:refnum<vi>)
  n121 = control-ref of="dw LP filter cut off frequency"() -> (w16:refnum<vi>)
  n122 = control-ref of="w12 LP  filter cutoff fequency"() -> (w17:refnum<vi>)
  n123 = control-ref of="w12 - dt"() -> (w20:refnum<vi>)
  n124 = control-ref of="w12 - a"() -> (w21:refnum<vi>)
  n125 = control-ref of="w12 - b"() -> (w22:refnum<vi>)
  n126 = control-ref of="Count to skip 5761, stage 1"() -> (w52:refnum<vi>)
  n127 = control-ref of="K2"() -> (w51:refnum<vi>)
  n128 = control-ref of="Q2"() -> (w50:refnum<vi>)
  n129 = control-ref of="w2"() -> (w49:refnum<vi>)
  n130 = control-ref of="K3"() -> (w48:refnum<vi>)
  n131 = control-ref of="Q3"() -> (w47:refnum<vi>)
  n132 = control-ref of="w3"() -> (w46:refnum<vi>)
  n133 = control-ref of="w0"() -> (w45:refnum<vi>)
  n134 = control-ref of="Output mixer fequency [MHz]"() -> (w76:refnum<vi>)
  n135 = control-ref of="Mixer freq [MHz]"() -> (w74:refnum<vi>)
  n136 = control-ref of="Transfer speed"() -> (w56:refnum<vi>)
  n137 = control-ref of="Piezo"() -> (w44:refnum<vi>)
  n138 = control-ref of="Output scale"() -> (w63:refnum<vi>)
  n139 = local write "Q0 identify"(w3) -> ()
  n140 = control-ref of="dw scale"() -> (w18:refnum<vi>)
  n141 = control-ref of="w12 scale"() -> (w19:refnum<vi>)
  n142 = control-ref of="Host scale"() -> (w61:refnum<vi>)
  n143 = control-ref of="Input scale"() -> (w60:refnum<vi>)
  n144 = control-ref of="Host scale 5761"() -> (w59:refnum<vi>)
  n145 = control-ref of="Input scale 5761"() -> (w58:refnum<vi>)
  n146 = local write "Rumode"(w3) -> ()
  n147 = control-ref of="Mode"() -> (w78:refnum<vi>)
  n148 = control-ref of="Trigger"() -> (w77:refnum<vi>)
  n149 = control-ref of="Output delay"() -> (w75:refnum<vi>)
  n150 = local write "Output enabled"(w122) -> ()
  n151 = local write "Zoom time Y"(w122) -> ()
  n152 = local write "Zoom time X"(w122) -> ()
  n153 = local write "Zoom freq X"(w122) -> ()
  n154 = local write "Zoom freq Y"(w122) -> ()
  n155 = local write "freqdata"(cluster{"f0":dbl, "df":dbl, "magnitude":dbl[]}[] [] ("freqdata")) -> ()
  n156 = local write "magnitude"(cluster{"f0":dbl, "df":dbl, "magnitude":dbl[]} {"f0"=0.0, "df"=0.0, "magnitude"=[]} ("magnitude")) -> ()
  n157 = property on="Tab Control" class="TabCtl (strict)"() -> ("Pages"=w41:refnum<vi>[])  [unwired: 2 in, 2 out]
  n158 = property on="Setpoint enabled" class="Bool (strict)"("Val(Sgnl)"=FALSE ("Value (Signaling)")) -> ()  [unwired: 2 in, 2 out]
  n159 = Bundle By Name(cluster="Graph_refs", "upper.Graph"=w138, "upper.Time btn"=w137, "upper.Amplitude btn"=w136, "upper.Chart"=w135, "lower.Graph"=w134, "lower.Time btn"=w133, "lower.Amplitude btn"=w132, "lower.Chart"=w131, "Freq graph"=w130, "Adaptive FF graph"=w110) -> (w71:T15)
  n160 = property on="Unwrap phase" class="Bool (strict)"("Val(Sgnl)"=TRUE ("Value (Signaling)")) -> ()  [unwired: 2 in, 2 out]
  n161 = flat-sequence {
    tunnel: [w197] -> w43
    frame #0 {
      w197 = FALSE
      w198 = fxp<+/-,32,6> 0.0 ("Kp")
      n162 = local write "Calculate w12"(w197) -> ()
      n163 = local write "Enable"(w197) -> ()
      n164 = property on="Hold plot lower" class="Bool (strict)"("Value"=w197) -> ()  [unwired: 2 in, 2 out]
      n165 = local write "Kp Q"(w198) -> ()
      n166 = local write "Kd/T  Q"(w198) -> ()
      n167 = local write "Kp AM"(w198) -> ()
      n168 = local write "Ki*T Q"(w198) -> ()
      n169 = local write "Kd/T AM"(w198) -> ()
      n170 = local write "Ki*T AM"(w198) -> ()
    }
  }
  n171 = for {
    tunnel: w41 -> [w204] mode=indexing
    tunnel: w25 -> [w199]
    n172 = case shown="True" w199 {
      tunnel: ["Quench" ("y") "Cavity model" ("y")] -> w202
      frame False {
      }
      frame True {
      }
    }
    n173 = property class="Page"(reference=w204) -> (reference out=w201:refnum<vi>, "PageLabel"=w203:string)  [unwired: 1 in, 1 out]
    n174 = Not Equal?(x=w203, y=w202) -> (x != y?=w200:bool)
    n175 = property class="Page"(reference=w201, "PageVis"=w200) -> ()  [unwired: 1 in, 2 out]
  }
  n176 = Current VI's Path() -> (path=w70:path)
  n177 = register-events(w127) -> (reference out=w144:refnum<event-registration>)  [unwired: 2 in, 1 out]
  n178 = Bundle By Name(cluster=w79, "Samples before reset"=w4, "Q0 - D"=w5, "Q0 - B"=w6, "Q0 - E"=w7, "Q0 - C"=w8, "Q0 - A"=w9, "sigm"=w10, "Nforget"=w11, "Vfi Vfq LP filter cut off frequency"=w12, "Vi Vq LP  filter cutoff fequency"=w13, "ch3 delay"=w14, "ch1 delay"=w15, "dw LP filter cut off frequency"=w16, "w12 LP  filter cutoff fequency"=w17, "dw scale"=w18, "w12 scale"=w19, "w12 - dt"=w20, "w12 - a"=w21, "w12 - b"=w22, "Mode"=w78, "Trigger"=w77, "Output mixer fequency [MHz]"=w76, "Output delay"=w75, "Mixer freq [MHz]"=w74, "Triggered"=w73, "Tranfer speed"=w56, "Continuous"=w72, "Output scale"=w63, "Host scale"=w61, "Input scale"=w60, "Host scale 5761"=w59, "Input scale 5761"=w58, "Virtual cavity"=w57, "Count to skip 5782, stage 1"=w53, "Count to skip 5761, stage 1"=w52, "K2"=w51, "Q2"=w50, "w2"=w49, "K3"=w48, "Q3"=w47, "w3"=w46, "w0"=w45, "Piezo"=w44, "Measure Tau at Time"=w40, "Tau set"=w39, "Count to skip 5761, stage 2"=w38, "Count to skip 5761, stage 3"=w37, "Count to skip 5782, stage 2"=w36, "Count to skip 5782, stage 3"=w35, "b"=w28, "a"=w27, "Fequency [kHz]"=w26) -> (w65:T3)
  "All FP controls" <- w65
  n179 = Open VI Reference(vi path=w70) -> (vi reference=w69:refnum<vi>)  [unwired: 5 in, 1 out]
  n180 = call "Init.vi"("vi reference"=w69, "Graph_refs"=w71, "SettingsFile in"=refnum<class "SettingsFileIQpid.lvclass"> refnum ("SettingsFileIQpid.lvclass")) -> ("Save event"=w67:T25, "SettingsFile out"=w66:refnum<class "SettingsFileIQpid.lvclass">)  [unwired: 6 in, 1 out]
  n181 = property on="Hold plot upper" class="Bool (strict)"("Val(Sgnl)"=w43) -> ()  [unwired: 2 in, 2 out]
  n182 = call "Init_IQ_PID.vi"("All FP controls"=w65, "SettingsFileIQpid in"=w66) -> ("SettingsFileIQpid out"=w23:refnum<class "SettingsFileIQpid.lvclass">)  [unwired: 8 in, 1 out]
  n183 = local write "Samples per 5782 record"(w121) -> ()
  n184 = local write "Mode"(w117) -> ()
  n185 = local write "Trigger"(w116) -> ()
  n186 = property class="VI"() -> ("Panel"=w55:refnum<vi>)  [unwired: 2 in, 2 out]
  n187 = control-ref of="Update once lower"() -> (w33:refnum<vi>)
  n188 = control-ref of="Update once upper"() -> (w34:refnum<vi>)
  n189 = case shown="No Error" w62 {
    tunnel: w111 -> [w219 w919]
    tunnel: [w218 w919] -> w113
    tunnel: w144 -> [w217 w918]
    tunnel: [w216 w918] -> w143
    tunnel: w71 -> [w214 _]
    tunnel: w121 -> [w213 _]
    tunnel: w67 -> [w212 _]
    tunnel: w55 -> [w211 w917]
    tunnel: [w210 w917] -> w54
    tunnel: w42 -> [w209 _]
    tunnel: w34 -> [w208 _]
    tunnel: w33 -> [w207 _]
    frame No Error {
      n190 = while {
        shift-right: [w228] -> w218
        shift-left: w219 -> [w235]
        tunnel: w217 -> [w233]
        tunnel: [w232] -> w216
        tunnel: [w231] -> w215
        tunnel: w214 -> [w230]
        tunnel: w213 -> [w229]
        tunnel: w212 -> [w226]
        shift-right: [w223] -> w210
        shift-left: w211 -> [w224]
        tunnel: w209 -> [w222]
        tunnel: w208 -> [w221]
        tunnel: w207 -> [w220]
        stop <- w231 stop-if-true
        n191 = call "GetTimeout.vi"("ScopeBase in"=w235) -> ("Time left"=w225:i32, "ScopeBase out"=w234:refnum<class "Scope5782_six_channel.lvclass">)  [unwired: 8 in, 1 out]
        n192 = event shown="[30] \"Singleshot\": Value Change" {
          selector: w233 -> [_ _ _ _ _ _ _ _ _ _ _ _ _ _ _ _ _ _ _ _ _ _ _ _ _ _ _ _ _ _ _ _ _ _ _ _ _ _ _ _ _ _ _ _ _ _ _ _ _ _ _ _ _ _ _ _ _ _ _ _ _ _ _ _ _]
          dyn-events: [_ _ _ _ _ _ _ _ _ _ _ _ _ _ _ _ _ _ _ _ _ _ _ _ _ _ _ _ _ _ _ _ _ _ _ _ _ _ _ _ _ _ _ _ _ _ _ _ _ _ _ _ _ _ _ _ _ _ _ _ _ _ _ _ _] -> w232
          timeout: w225 -> [_ _ _ _ _ _ _ _ _ _ _ _ _ _ _ _ _ _ _ _ _ _ _ _ _ _ _ _ _ _ _ _ _ _ _ _ _ _ _ _ _ _ _ _ _ _ _ _ _ _ _ _ _ _ _ _ _ _ _ _ _ _ _ _ _]
          tunnel: [_ w295 _ _ _ _ _ _ _ _ _ _ _ _ _ _ _ _ _ _ _ _ _ _ _ _ _ _ _ _ _ _ _ "stop" _ _ _ _ _ _ _ _ _ _ _ _ _ _ _ _ _ _ _ _ _ _ _ _ _ _ _ _ _ _ _] -> w231
          tunnel: w234 -> [w263 w297 w308 w323 w326 w333 w343 w368 w388 w416 w422 w436 w442 w448 w454 w460 w466 w475 w479 w485 w489 w502 w518 w520 w532 w542 w549 w554 w570 w608 w610 w616 w626 w628 w636 w648 w654 w662 w674 w682 w688 w698 w710 w716 w728 w734 w740 w744 w751 w758 w760 w767 w773 w779 w786 w805 w811 w832 w845 w854 w861 w864 w894 w900 w914]
          tunnel: [w252 w297 w308 w321 w325 w330 w342 w367 w387 w415 w420 w432 w441 w447 w453 w459 w465 w469 w478 w484 w490 w503 w517 w521 w531 w541 w547 w552 w565 w606 w611 w614 w626 w628 w636 w648 w654 w662 w674 w678 w686 w697 w709 w715 w727 w733 w739 w743 w750 w757 w759 w766 w772 w778 w785 w803 w809 w818 w844 w851 w860 w863 w893 w899 w915] -> w228
          tunnel: w230 -> [_ _ _ _ _ _ _ _ _ _ _ _ _ _ _ _ _ _ _ _ _ _ _ _ _ _ _ _ w559 _ _ _ _ _ _ _ _ _ w672 _ _ _ _ _ _ _ _ _ _ _ _ _ _ _ _ _ _ _ _ _ _ _ _ _ _]
          tunnel: w229 -> [_ _ _ _ _ _ _ _ _ _ _ _ _ _ _ _ _ _ _ _ _ _ _ _ _ _ _ _ w568 _ _ _ _ _ _ _ _ _ _ _ _ _ _ _ _ _ _ _ _ _ _ _ _ _ _ _ _ _ _ _ _ _ _ _ _]
          tunnel: w226 -> [_ w294 _ _ _ _ _ _ _ _ _ _ _ _ _ _ _ _ _ _ _ _ _ _ _ _ _ _ _ _ _ _ _ _ _ _ _ _ _ _ _ _ _ _ _ _ _ _ _ _ _ _ _ _ _ _ _ _ _ _ _ _ _ _ _]
          tunnel: [TRUE _ _ _ _ _ _ _ _ _ _ _ _ _ _ _ _ _ _ _ _ _ _ _ _ _ _ _ _ _ _ _ _ _ _ _ _ _ _ _ _ _ _ _ _ _ _ _ _ _ _ _ _ _ _ _ _ _ _ _ _ _ _ _ _] -> w227
          tunnel: [w240 w293 w304 w320 w324 w329 w348 w359 w379 w414 w431 w437 w438 w444 w450 w456 w462 w468 w477 w483 w487 w500 w513 w519 w528 w537 w546 w551 w564 w605 w609 w615 w624 w627 w630 w640 w649 w655 w666 w677 w685 w693 w705 w711 w723 w729 w735 w741 w747 w753 w764 w770 w776 w782 w800 w806 w816 w841 w850 w855 w862 w886 w897 w901 w916] -> w223
          tunnel: w224 -> [w250 w293 w304 w320 w324 w329 w348 w359 w379 w414 w431 w437 w438 w444 w450 w456 w462 w468 w477 w483 w487 w500 w513 w519 w528 w537 w546 w551 w564 w605 w609 w615 w624 w627 w630 w640 w649 w655 w666 w677 w685 w693 w705 w711 w723 w729 w735 w741 w747 w753 w764 w770 w776 w782 w800 w806 w816 w841 w850 w855 w862 w886 w897 w901 w916]
          tunnel: w222 -> [w264 _ _ _ _ _ _ _ _ _ _ _ _ _ _ _ _ _ _ _ _ _ _ _ _ _ _ _ _ _ _ _ _ _ _ _ _ _ _ _ _ _ _ _ _ _ _ _ _ _ _ _ _ _ _ _ _ _ _ _ _ _ _ _ _]
          tunnel: w221 -> [w261 _ _ _ _ _ _ _ _ _ _ _ _ _ _ _ _ _ _ _ _ _ _ _ _ _ _ _ _ _ _ _ _ _ _ _ _ _ _ _ _ _ _ _ _ _ _ _ _ _ _ _ _ _ _ _ _ _ _ _ _ _ _ _ _]
          tunnel: w220 -> [w262 _ _ _ _ _ _ _ _ _ _ _ _ _ _ _ _ _ _ _ _ _ _ _ _ _ _ _ _ _ _ _ _ _ _ _ _ _ _ _ _ _ _ _ _ _ _ _ _ _ _ _ _ _ _ _ _ _ _ _ _ _ _ _ _]
          event Timeout {
            n193 = event-data() -> ()  [unwired: 1 in, 3 out]
            n194 = local read "Reference for phase"() -> (w260:T14)
            n195 = local read "Transfer speed"() -> (w258:T2)
            n196 = local read "Unwrap phase"() -> (w256:bool)
            n197 = property class="Pnl"(reference=w250, "DeferPanUpdts"=TRUE ("Defer Panel Updates")) -> (reference out=w243:refnum<vi>)  [unwired: 1 in, 1 out]
            n198 = local read "Window"() -> (w255:T13)
            n199 = local read "Display"() -> (w254:T18)
            n200 = local read "Buffer"() -> (w253:T17)
            n201 = local read "#bins"() -> (w259:i32)
            n202 = local read "Unit"() -> (w257:T12)
            n203 = call "AddDataToPlots.vi"("Scope5761 in"=w263, "Display"=w254, "Buffer"=w253, "Unwrap phase"=w256, "Transfer speed"=w258, "Reference for phase"=w260, "Window"=w255, "Unit"=w257, "#bins"=w259, "Update once lower"=w262, "Update once upper"=w261) -> ("Uppder data"=w247:dbl[][], "magnitude out"=w238:cluster{"f0":dbl, "df":dbl, "magnitude":dbl[]}, "Lower data"=w245:dbl[][], "Scope5761 out"=w252:refnum<class "Scope5782_six_channel.lvclass">, "Freqdata"=w244:cluster{"f0":dbl, "df":dbl, "magnitude":dbl[]}[], "Any read?"=w251:bool, "Write upper"=w248:T30, "Write lower"=w246:T30)  [unwired: 9 in]
            n204 = local read "quench"() -> (w239:bool)
            n205 = case shown="\"Graph\"" w248 {
              selector: w248 -> [_ _ w292]
              tunnel: w247 -> [w290 w291 _]
              tunnel: [_ _ w292] -> w241
              frame "Graph" {
                "Upper graph" <- w290
              }
              frame "Chart" {
                "Upper chart" <- w291
              }
              frame "None", Default {
              }
            }
            n206 = case shown="\"Freq\"" w246 {
              selector: w246 -> [w285 _ _ _]
              tunnel: w245 -> [_ w286 w287 _]
              tunnel: w244 -> [_ _ _ w289]
              tunnel: [w285 _ _ _] -> w242
              tunnel: w238 -> [_ _ _ w288]
              frame "None", Default {
              }
              frame "Graph" {
                "Lower graph" <- w286
              }
              frame "Chart" {
                "Lower chart" <- w287
              }
              frame "Freq" {
                "freqdata" <- w289
                "magnitude" <- w288
              }
            }
            n207 = case shown="True" w239 {
              tunnel: w264 -> [_ w267]
              tunnel: w251 -> [_ w266]
              frame False {
              }
              frame True {
                n208 = case shown="True" w266 {
                  tunnel: w267 -> [_ w277]
                  frame False {
                  }
                  frame True {
                    n209 = xnode "Read/Write Control"("FPGA VI Reference In"=w277) -> ("FPGA VI Reference Out"=w269:refnum<k20>, "Quench_Warning"=w272:bool, "Amp1"=→"Amp1":fxp<+,16,14>, "TaM"=w275:fxp<+/-,32,13>, "Tau_set"=→"Tau_set":fxp<+/-,32,13>)  [unwired: 1 in, 1 out]
                    "Quench_Warning" <- w272
                    n210 = local read "Reset Quench Warning"() -> (w273:bool)
                    n211 = Compound Arithmetic op=AND(w273, invert w272) -> (w271:bool)
                    n212 = case shown="True" w271 {
                      tunnel: w269 -> [_ w281]
                      frame False {
                      }
                      frame True {
                        n213 = local write "Reset Quench Warning"(FALSE ("Reset Quench Warning")) -> ()
                        n214 = call "Write 16bit value.vi"("value"=fxp<+,16,16> 0.0, "FPGA Setting"=fpga_settings."Quench reset", "FPGA ref"=w281) -> ()  [unwired: 7 in, 2 out]
                      }
                    }
                    n215 = Multiply(x=w275, y=fxp<+/-,32,13> 6.399999618530273 ("x")) -> (x*y=→"Tau [µs]":fxp<+/-,64,26>)
                  }
                }
              }
            }
            n216 = flat-sequence {
              tunnel: w243 -> [w283]
              tunnel: w242 -> [_]
              tunnel: w241 -> [_]
              tunnel: [w282] -> w240
              frame #0 {
                n217 = property class="Pnl"(reference=w283, "DeferPanUpdts"=FALSE ("Defer Panel Updates")) -> (reference out=w282:refnum<vi>)  [unwired: 1 in, 1 out]
              }
            }
          }
          event Menu Selection (User) {
            n218 = event-data() -> ("ItemTag"=w296:string)  [unwired: 1 in, 6 out]
            n219 = case shown="\"Quit\"" w296 {
              tunnel: [_ w298 _ _] -> w295
              tunnel: w294 -> [_ _ w301 w303]
              frame "False", Default {
              }
              frame "Quit" {
                n220 = Two Button Dialog(message="Exit application?") -> (T button?=w298:bool)  [unwired: 2 in]
              }
              frame "SaveSettings" {
                n221 = Generate User Event(user event=w301, event data cluster=T26 {"Automatic"=FALSE, "Save"=TRUE} ("event data")) -> ()  [unwired: 2 in, 2 out]
              }
              frame "LoadSettings" {
                n222 = Generate User Event(user event=w303, event data cluster=T26 {"Automatic"=FALSE, "Save"=FALSE} ("event data")) -> ()  [unwired: 2 in, 2 out]
              }
            }
          }
          event Value Change {
            n223 = event-data() -> ("OldVal"=w305:T14)  [unwired: 1 in, 5 out]
            n224 = local read "Display"() -> (w306:T18)
            n225 = case shown="\"Phase and Magnitude\"" w306 {
              tunnel: "Reference for phase" -> [_ w313]
              tunnel: w305 -> [_ w311]
              frame "Time and Frequency", Default {
              }
              frame "Phase and Magnitude" {
                n226 = property on="Lower chart" class="WFChart (strict)"() -> ("History Data"=w312:dbl[][])  [unwired: 2 in, 2 out]
                n227 = Index Array(array=w312, index (row)=w311) -> (element=w310:dbl[])  [unwired: 1 in]
                n228 = Index Array(array=w312, index (row)=w313) -> (element=w314:dbl[])  [unwired: 1 in]
                n229 = for {
                  tunnel: w312 -> [w317] mode=indexing
                  tunnel: w314 -> [w319]
                  tunnel: [w318] -> w309 mode=indexing
                  tunnel: w310 -> [w316] mode=indexing
                  n230 = Add(x=w317, y=w316) -> (x+y=w315:dbl[])
                  n231 = Subtract(x=w315, y=w319) -> (x-y=w318:dbl[])
                }
                n232 = property on="Lower chart" class="WFChart (strict)"("History Data"=w309) -> ()  [unwired: 2 in, 2 out]
              }
            }
          }
          event "Mixer freq [MHz]": Value Change {
            n233 = event-data() -> ()  [unwired: 1 in, 6 out]
            n234 = call-dynamic "SetMixerFrequency.vi"("Mixer freq [MHz]"="Mixer freq [MHz]", "Scope5785_six_channel"=w323) -> ("Scope5785_six_channel Out"=w321:refnum<class "Scope5782_six_channel.lvclass">)  [unwired: 8 in, 1 out]
          }
          event "Fequency [MHz]", "Phase offset (deg)": Value Change {
            n235 = event-data() -> ()  [unwired: 1 in, 6 out]
            n236 = call-dynamic "SetSimulatedFreq.vi"("Phase offset (deg)"="Phase offset (deg)", "Mixer freq [MHz]"="Fequency [MHz]", "Scope5785_six_channel"=w326) -> ("Scope5785_six_channel out"=w325:refnum<class "Scope5782_six_channel.lvclass">)  [unwired: 7 in, 1 out]
          }
          event "Output mixer fequency [MHz]", "Output enabled": Value Change {
            n237 = event-data() -> ()  [unwired: 1 in, 6 out]
            n238 = call "SetOutputFreq.vi"("Output enabled"="Output enabled", "Output mixer fequency [MHz]"="Output mixer fequency [MHz]", "Scope5785_six_channel"=w333) -> ("Scope5785_six_channel out"=w330:refnum<class "Scope5782_six_channel.lvclass">)  [unwired: 7 in, 1 out]
          }
          event "Output delay", "Output delay delta": Value Change {
            w345 = fxp<+/-,16,2> 0.0 ("x")
            n239 = event-data() -> ()  [unwired: 1 in, 6 out]
            n240 = local read "Mixer freq [MHz]"() -> (w351:dbl)
            n241 = Multiply(x="Output delay", y=0.001) -> (x*y=w352:dbl)
            n242 = Multiply(x="Output delay delta", y=1e-06) -> (x*y=w354:dbl)
            n243 = call "Read FpgaRef5782.vi"("Scope5785_six_channel"=w343) -> ("FpgaRef5782.lvclass"=w341:refnum<class "FpgaRef5782.lvclass">, "Scope5785_six_channel Out"=w342:refnum<class "Scope5782_six_channel.lvclass">)  [unwired: 8 in, 1 out]
            n244 = Multiply(x=w351, y=6.283185307179586) -> (x*y=w349:dbl)
            n245 = Multiply(x=w349, y=w354) -> ()  [unwired: 1 out]
            n246 = Multiply(x=w352, y=w349) -> (x*y=w340:dbl)
            n247 = Sine & Cosine(0:w340) -> (1:w346:dbl, 2:w344:dbl)
            n248 = To Fixed-Point(fixed-point type=w345, number=w346) -> (fixed-point=w347:fxp<+/-,16,2>)
            n249 = To Fixed-Point(fixed-point type=w345, number=w344) -> (fixed-point=w339:fxp<+/-,16,2>)
            n250 = xnode "Reinterpret Number"("x"=w347) -> ("y"=w338:fxp<+,16,16>)
            n251 = xnode "Reinterpret Number"("x"=w339) -> ("y"=w337:fxp<+,16,16>)
            n252 = call "WriteSetting 16bit.vi"("value"=w338, "FPGA Setting"=fpga_settings."fixed sin_fi", "FpgaRefBase in"=w341) -> ("FpgaRefBase out"=w336:refnum<class "FpgaRef5782.lvclass">)  [unwired: 7 in, 1 out]
            n253 = call "WriteSetting 16bit.vi"("value"=w337, "FPGA Setting"=fpga_settings."fixed cos_fi", "FpgaRefBase in"=w336) -> ()  [unwired: 7 in, 2 out]
          }
          event "Ki*T AM", "Kd/T AM", "Kp AM": Value Change {
            n254 = event-data() -> ()  [unwired: 1 in, 6 out]
            n255 = xnode "Reinterpret Number"("x"="Kd/T AM") -> ("y"=w376:fxp<+,32,32>)
            n256 = xnode "Reinterpret Number"("x"="Ki*T AM") -> ("y"=w375:fxp<+,32,32>)
            n257 = xnode "Reinterpret Number"("x"="Kp AM") -> ("y"=w377:fxp<+,32,32>)
            n258 = To Unsigned Long Integer(number=w375) -> (unsigned 32bit integer=w362:u32)
            n259 = To Unsigned Long Integer(number=w376) -> (unsigned 32bit integer=w361:u32)
            n260 = To Unsigned Long Integer(number=w377) -> (unsigned 32bit integer=w360:u32)
            n261 = call "Write Setting 16bit.vi"("value"="I Feedback", "FPGA Setting"=fpga_settings."PID enabled I", "ScopeBase in"=w368) -> ("ScopeBase out"=w371:refnum<class "Scope5782_six_channel.lvclass">)  [unwired: 7 in, 1 out]
            n262 = call "Write Setting 32bit.vi"("value"=w362, "FPGA Setting"=fpga_settings."Ki*Tau am", "ScopeBase in"=w371) -> ("ScopeBase out"=w370:refnum<class "Scope5782_six_channel.lvclass">)  [unwired: 7 in, 1 out]
            n263 = call "Write Setting 32bit.vi"("value"=w361, "FPGA Setting"=fpga_settings."Kd_Tau am", "ScopeBase in"=w370) -> ("ScopeBase out"=w369:refnum<class "Scope5782_six_channel.lvclass">)  [unwired: 7 in, 1 out]
            n264 = call "Write Setting 32bit.vi"("value"=w360, "FPGA Setting"=fpga_settings."Kp am", "ScopeBase in"=w369) -> ("ScopeBase out"=w367:refnum<class "Scope5782_six_channel.lvclass">)  [unwired: 7 in, 1 out]
          }
          event "Kp Q", "Kd/T  Q", "Ki*T Q": Value Change {
            n265 = event-data() -> ()  [unwired: 1 in, 6 out]
            n266 = xnode "Reinterpret Number"("x"="Kd/T  Q") -> ("y"=w396:fxp<+,32,32>)
            n267 = xnode "Reinterpret Number"("x"="Ki*T Q") -> ("y"=w395:fxp<+,32,32>)
            n268 = xnode "Reinterpret Number"("x"="Kp Q") -> ("y"=w397:fxp<+,32,32>)
            n269 = To Unsigned Long Integer(number=w395) -> (unsigned 32bit integer=w382:u32)
            n270 = To Unsigned Long Integer(number=w396) -> (unsigned 32bit integer=w381:u32)
            n271 = To Unsigned Long Integer(number=w397) -> (unsigned 32bit integer=w380:u32)
            n272 = call "Write Setting 16bit.vi"("value"="Q Feedback", "FPGA Setting"=fpga_settings."Feedback Enable", "ScopeBase in"=w388) -> ("ScopeBase out"=w391:refnum<class "Scope5782_six_channel.lvclass">)  [unwired: 7 in, 1 out]
            n273 = call "Write Setting 32bit.vi"("value"=w382, "FPGA Setting"=fpga_settings."Ki*Tau Q", "ScopeBase in"=w391) -> ("ScopeBase out"=w390:refnum<class "Scope5782_six_channel.lvclass">)  [unwired: 7 in, 1 out]
            n274 = call "Write Setting 32bit.vi"("value"=w381, "FPGA Setting"=fpga_settings."Kd_Tau Q", "ScopeBase in"=w390) -> ("ScopeBase out"=w389:refnum<class "Scope5782_six_channel.lvclass">)  [unwired: 7 in, 1 out]
            n275 = call "Write Setting 32bit.vi"("value"=w380, "FPGA Setting"=fpga_settings."Kp Q", "ScopeBase in"=w389) -> ("ScopeBase out"=w387:refnum<class "Scope5782_six_channel.lvclass">)  [unwired: 7 in, 1 out]
          }
          event "w12", "R1", "w1", "Q1", "K1", "S", "K2", "Q2", "w2", "K3", "Q3", "w3": Value Change {
            n276 = event-data() -> ()  [unwired: 1 in, 6 out]
            n277 = call "CavityConstanstToFIFO.vi"("w12"="w12", "Mechanical mode"=1, "R1"="R1", "w1"="w1", "Q1"="Q1", "K1"="K1", "S"="S") -> ("FIFO array"=w413:u64[])  [unwired: 8 in]
            n278 = call "CavityConstanstToFIFO.vi"("w12"="w12", "Mechanical mode"=2, "R1"="R1", "w1"="w2", "Q1"="Q2", "K1"="K2", "S"="S") -> ("FIFO array"=w411:u64[])  [unwired: 8 in]
            n279 = call "CavityConstanstToFIFO.vi"("w12"="w12", "Mechanical mode"=3, "R1"="R1", "w1"="w3", "Q1"="Q3", "K1"="K3", "S"="S") -> ("FIFO array"=w398:u64[])  [unwired: 8 in]
            n280 = Build Array (concatenate)(w413, w411, w398) -> (w412:u64[])
            n281 = call "Write Setting Array.vi"("Data"=w412, "ScopeBase in"=w416) -> ("ScopeBase out"=w415:refnum<class "Scope5782_six_channel.lvclass">)  [unwired: 8 in, 1 out]
          }
          event "w0": Value Change {
            w425 = 1e-07  # dt
            n282 = event-data() -> ()  [unwired: 1 in, 6 out]
            n283 = Multiply(x="w0", y=w425) -> (x*y=w424:dbl)
            n284 = To Fixed-Point(fixed-point type=fxp<+/-,48,0> 0.0 ("x"), number=w424) -> (fixed-point=w430:fxp<+/-,48,0>)
            n285 = xnode "Reinterpret Number"("x"=w430) -> ("y"=w428:fxp<+,48,48>)
            n286 = call "To48BitSetting.vi"("48 bit value"=w428, "FPGA Setting"=fpga_settings."Cavity_w0_dt") -> ("value"=w423:u64)  [unwired: 9 in]
            n287 = Build Array(w423) -> (w421:u64[])
            n288 = call "Write Setting Array.vi"("Data"=w421, "ScopeBase in"=w422) -> ("ScopeBase out"=w420:refnum<class "Scope5782_six_channel.lvclass">)  [unwired: 8 in, 1 out]
          }
          event Value Change {
            n289 = event-data() -> ()  [unwired: 1 in, 6 out]
            n290 = To Unsigned Long Integer(number="Piezo") -> (unsigned 32bit integer=w433:u32)
            n291 = call "Write Setting 32bit.vi"("value"=w433, "FPGA Setting"=fpga_settings."Piezo setting", "ScopeBase in"=w436) -> ("ScopeBase out"=w432:refnum<class "Scope5782_six_channel.lvclass">)  [unwired: 7 in, 1 out]
          }
          event "ch0 DC offset": Value Change {
            n292 = event-data() -> ()  [unwired: 1 in, 6 out]
            n293 = call "Read FpgaRef5782.vi"("Scope5785_six_channel"=w442) -> ("FpgaRef5782.lvclass"=w443:refnum<class "FpgaRef5782.lvclass">, "Scope5785_six_channel Out"=w441:refnum<class "Scope5782_six_channel.lvclass">)  [unwired: 8 in, 1 out]
            n294 = call "SetDcOffset.vi"("FPGA Setting"=fpga_settings."DC_offs 0", "DC offset"="ch0 DC offset", "FpgaRef5782 in"=w443) -> ()  [unwired: 7 in, 2 out]
          }
          event "ch0 DC offset 2": Value Change {
            n295 = event-data() -> ()  [unwired: 1 in, 6 out]
            n296 = call "Read FpgaRef5761.vi"("Scope5785_six_channel"=w448) -> ("FpgaRef5761.lvclass"=w449:refnum<class "FpgaRef5761.lvclass">, "Scope5785_six_channel Out"=w447:refnum<class "Scope5782_six_channel.lvclass">)  [unwired: 8 in, 1 out]
            n297 = call "SetDcOffset.vi"("FPGA Setting"=fpga_settings."DC_offs 0", "DC offset"="ch0 DC offset 2", "FpgaRef5761 In"=w449) -> ()  [unwired: 7 in, 2 out]
          }
          event "ch1 DC offset 2": Value Change {
            n298 = event-data() -> ()  [unwired: 1 in, 6 out]
            n299 = call "Read FpgaRef5761.vi"("Scope5785_six_channel"=w454) -> ("FpgaRef5761.lvclass"=w455:refnum<class "FpgaRef5761.lvclass">, "Scope5785_six_channel Out"=w453:refnum<class "Scope5782_six_channel.lvclass">)  [unwired: 8 in, 1 out]
            n300 = call "SetDcOffset.vi"("FPGA Setting"=fpga_settings."DC_offs 1", "DC offset"="ch1 DC offset 2", "FpgaRef5761 In"=w455) -> ()  [unwired: 7 in, 2 out]
          }
          event "ch2 DC offset": Value Change {
            n301 = event-data() -> ()  [unwired: 1 in, 6 out]
            n302 = call "Read FpgaRef5761.vi"("Scope5785_six_channel"=w460) -> ("FpgaRef5761.lvclass"=w461:refnum<class "FpgaRef5761.lvclass">, "Scope5785_six_channel Out"=w459:refnum<class "Scope5782_six_channel.lvclass">)  [unwired: 8 in, 1 out]
            n303 = call "SetDcOffset.vi"("FPGA Setting"=fpga_settings."DC_offs 2", "DC offset"="ch2 DC offset", "FpgaRef5761 In"=w461) -> ()  [unwired: 7 in, 2 out]
          }
          event "ch3 DC offset": Value Change {
            n304 = event-data() -> ()  [unwired: 1 in, 6 out]
            n305 = call "Read FpgaRef5761.vi"("Scope5785_six_channel"=w466) -> ("FpgaRef5761.lvclass"=w467:refnum<class "FpgaRef5761.lvclass">, "Scope5785_six_channel Out"=w465:refnum<class "Scope5782_six_channel.lvclass">)  [unwired: 8 in, 1 out]
            n306 = call "SetDcOffset.vi"("FPGA Setting"=fpga_settings."DC_offs 3", "DC offset"="ch3 DC offset", "FpgaRef5761 In"=w467) -> ()  [unwired: 7 in, 2 out]
          }
          event "Feedback delay", "Trigger delay": Value Change {
            n307 = event-data() -> ()  [unwired: 1 in, 6 out]
            n308 = Add(x="Feedback delay", y="Trigger delay") -> (x+y=w473:u32)
            n309 = call "Write Setting 32bit.vi"("value"=w473, "FPGA Setting"=fpga_settings."Feedback delay", "ScopeBase in"=w475) -> ("ScopeBase out"=w471:refnum<class "Scope5782_six_channel.lvclass">)  [unwired: 7 in, 1 out]
            n310 = call "Write Setting 32bit.vi"("value"="Trigger delay", "FPGA Setting"=fpga_settings."Trigger delay", "ScopeBase in"=w471) -> ("ScopeBase out"=w469:refnum<class "Scope5782_six_channel.lvclass">)  [unwired: 7 in, 1 out]
          }
          event "Acquire samples": Value Change {
            n311 = event-data() -> ()  [unwired: 1 in, 6 out]
            n312 = call "Write Setting 32bit.vi"("value"="Acquire samples", "FPGA Setting"=fpga_settings."Samples to acquire", "ScopeBase in"=w479) -> ("ScopeBase out"=w478:refnum<class "Scope5782_six_channel.lvclass">)  [unwired: 7 in, 1 out]
          }
          event "Samples before reset": Value Change {
            n313 = event-data() -> ()  [unwired: 1 in, 6 out]
            n314 = call "Write Setting 32bit.vi"("value"="Samples before reset", "FPGA Setting"=fpga_settings."Samples before reset", "ScopeBase in"=w485) -> ("ScopeBase out"=w484:refnum<class "Scope5782_six_channel.lvclass">)  [unwired: 7 in, 1 out]
          }
          event "show setpoint": Value Change {
            n315 = event-data() -> ()  [unwired: 1 in, 6 out]
            n316 = call "Read Feedforward.vi"("Scope5785_six_channel"=w489) -> ("Feeforward"=w488:T31, "Scope5785_six_channel out"=w490:refnum<class "Scope5782_six_channel.lvclass">)  [unwired: 8 in, 1 out]
            n317 = Unbundle By Name(w488) -> ("Setpoint I"=w497:dbl[], "Setpoint Q"=w496:dbl[])
            n318 = Array Size(array=w497) -> (size(s)=w495:i32)
            n319 = Array Size(array=w496) -> (size(s)=w494:i32)
            n320 = Build Array(w497, w496) -> (w498:dbl[][])
            n321 = Greater Than 0?(x=w495) -> (x > 0?=w493:bool)
            n322 = Greater Than 0?(x=w494) -> (x > 0?=w492:bool)
            n323 = And(x=w493, y=w492) -> (x .and. y?=w491:bool)
            n324 = case shown="True" w491 {
              tunnel: w498 -> [_ w499]
              frame False {
              }
              frame True {
                n325 = call "ShowIQvaluesAsync.vi"("IQ data"=w499) -> ()  [unwired: 11 in]
              }
            }
          }
          event "show feedforward": Value Change {
            n326 = event-data() -> ()  [unwired: 1 in, 6 out]
            n327 = call "Read Feedforward.vi"("Scope5785_six_channel"=w502) -> ("Feeforward"=w501:T31, "Scope5785_six_channel out"=w503:refnum<class "Scope5782_six_channel.lvclass">)  [unwired: 8 in, 1 out]
            n328 = Unbundle By Name(w501) -> ("Feedforward I"=w510:dbl[], "Feedforward Q"=w509:dbl[])
            n329 = Array Size(array=w510) -> (size(s)=w508:i32)
            n330 = Array Size(array=w509) -> (size(s)=w507:i32)
            n331 = Build Array(w510, w509) -> (w511:dbl[][])
            n332 = Greater Than 0?(x=w508) -> (x > 0?=w506:bool)
            n333 = Greater Than 0?(x=w507) -> (x > 0?=w505:bool)
            n334 = And(x=w506, y=w505) -> (x .and. y?=w504:bool)
            n335 = case shown="True" w504 {
              tunnel: w511 -> [_ w512]
              frame False {
              }
              frame True {
                n336 = call "ShowIQvaluesAsync.vi"("IQ data"=w512) -> ()  [unwired: 11 in]
              }
            }
          }
          event "ch1 DC offset": Value Change {
            n337 = event-data() -> ()  [unwired: 1 in, 6 out]
            n338 = call "Read FpgaRef5782.vi"("Scope5785_six_channel"=w518) -> ("FpgaRef5782.lvclass"=w516:refnum<class "FpgaRef5782.lvclass">, "Scope5785_six_channel Out"=w517:refnum<class "Scope5782_six_channel.lvclass">)  [unwired: 8 in, 1 out]
            n339 = call "SetDcOffset.vi"("FPGA Setting"=fpga_settings."DC_offs 1", "DC offset"="ch1 DC offset", "FpgaRef5782 in"=w516) -> ()  [unwired: 7 in, 2 out]
          }
          event "Setpoint enabled": Value Change {
            n340 = event-data() -> ()  [unwired: 1 in, 6 out]
            n341 = Boolean To (0,1)(Boolean="Setpoint enabled") -> (0, 1=w524:i16)
            n342 = To Word Integer(number=w524) -> (16bit integer=w526:i16)
            n343 = xnode "Reinterpret Number"("x"=w526) -> ("y"=w527:fxp<+/-,16,14>)
            n344 = xnode "Reinterpret Number"("x"=w527) -> ("y"=w523:fxp<+,16,16>)
            n345 = call "Write Setting 16bit.vi"("value"=w523, "FPGA Setting"=fpga_settings."Setpoint enable", "ScopeBase in"=w520) -> ("ScopeBase out"=w521:refnum<class "Scope5782_six_channel.lvclass">)  [unwired: 7 in, 1 out]
          }
          event "Cavity model": Value Change {
            n346 = event-data() -> ()  [unwired: 1 in, 6 out]
            n347 = Boolean To (0,1)(Boolean="Cavity model") -> (0, 1=w534:i16)
            n348 = To Word Integer(number=w534) -> (16bit integer=w535:i16)
            n349 = xnode "Reinterpret Number"("x"=w535) -> ("y"=w536:fxp<+/-,16,14>)
            n350 = xnode "Reinterpret Number"("x"=w536) -> ("y"=w529:fxp<+,16,16>)
            n351 = call "Write Setting 16bit.vi"("value"=w529, "FPGA Setting"=fpga_settings."Cavity Enable", "ScopeBase in"=w532) -> ("ScopeBase out"=w531:refnum<class "Scope5782_six_channel.lvclass">)  [unwired: 7 in, 1 out]
          }
          event "Virtual cavity": Value Change {
            n352 = event-data() -> ()  [unwired: 1 in, 6 out]
            n353 = Boolean To (0,1)(Boolean="Virtual cavity") -> (0, 1=w543:i16)
            n354 = To Word Integer(number=w543) -> (16bit integer=w544:i16)
            n355 = xnode "Reinterpret Number"("x"=w544) -> ("y"=w545:fxp<+/-,16,14>)
            n356 = xnode "Reinterpret Number"("x"=w545) -> ("y"=w539:fxp<+,16,16>)
            n357 = call "Write Setting 16bit.vi"("value"=w539, "FPGA Setting"=fpga_settings."Virtual cavity", "ScopeBase in"=w542) -> ("ScopeBase out"=w541:refnum<class "Scope5782_six_channel.lvclass">)  [unwired: 7 in, 1 out]
          }
          event Value Change {
            n358 = event-data() -> ()  [unwired: 1 in, 6 out]
            n359 = property on="Rumode" class="Bool (strict)"("Val(Sgnl)"=FALSE ("Value (Signaling)")) -> ()  [unwired: 2 in, 2 out]
            n360 = call-dynamic "SetMode.vi"("Mode"="Mode", "ScopeBase In"=w549) -> ("ScopeBase Out"=w547:refnum<class "Scope5782_six_channel.lvclass">)  [unwired: 8 in, 1 out]
          }
          event Value Change {
            n361 = event-data() -> ()  [unwired: 1 in, 6 out]
            n362 = call-dynamic "SetTrigger.vi"("Trigger"="Trigger", "ScopeBase In"=w554) -> ("ScopeBase Out"=w552:refnum<class "Scope5782_six_channel.lvclass">)  [unwired: 8 in, 1 out]
          }
          event Value Change {
            w572 = dbl[][] [] ("History Data")
            n363 = event-data() -> ()  [unwired: 1 in, 6 out]
            n364 = case shown="\"Very high speed (10Ms/s)\"" "Transfer speed" {
              tunnel: [w580 w586 w594 w602] -> w567
              tunnel: w568 -> [w581 w589 w597 w602]
              tunnel: [0.0001 ("t") 0.02 ("t") 0.05 ("t") 0.001 ("t")] -> w560
              tunnel: [T28."Disabled and Grayed Out" ("Disabled") T28."Enabled" ("Disabled") T28."Enabled" ("Disabled") T28."Disabled and Grayed Out" ("Disabled")] -> w563
              tunnel: [6 ("dimension size") 14 ("dimension size") 14 ("dimension size") 14 ("dimension size")] -> w561
              frame "Very high speed (10Ms/s)" {
                n365 = Multiply(x=10, y=w581) -> (x*y=w580:i32)
              }
              frame "Low speed (50kS/s)" {
                n366 = Divide(x=w589, y=20 ("x")) -> (x/y=w588:dbl)
                n367 = Round To Nearest(number=w588) -> (nearest integer value=w587:dbl)
                n368 = To Long Integer(number=w587) -> (32bit integer=w586:i32)
              }
              frame "Ultra low speed (20kS/s)" {
                n369 = Divide(x=w597, y=50 ("x")) -> (x/y=w596:dbl)
                n370 = Round To Nearest(number=w596) -> (nearest integer value=w595:dbl)
                n371 = To Long Integer(number=w595) -> (32bit integer=w594:i32)
              }
              frame "High speed (1Ms/s)" {
              }
            }
            n372 = property on="FFT buffer size" class="Enum (strict)"("DisabledEnum"=w563) -> ()  [unwired: 2 in, 2 out]
            n373 = call-dynamic "SetRecordLength.vi"("Samples per 5782 record"=w567, "ScopeBase In"=w570) -> ("ScopeBase Out"=w569:refnum<class "Scope5782_six_channel.lvclass">)  [unwired: 8 in, 1 out]
            n374 = property on="Lower chart" class="WFChart (strict)"("History Data"=w572) -> ()  [unwired: 2 in, 2 out]
            n375 = property on="Upper chart" class="WFChart (strict)"("History Data"=w572) -> (error out=w573:errorcluster)  [unwired: 2 in, 1 out]
            n376 = Initialize Array(nan ("element"), 4 ("dimension size"), w567) -> (w575:dbl[][])
            n377 = call-dynamic "SetFullSpeedTransfer.vi"("Tranfer speed"="Transfer speed", "ScopeBase In"=w569) -> ("ScopeBase Out"=w566:refnum<class "Scope5782_six_channel.lvclass">)  [unwired: 8 in, 1 out]
            n378 = local read "Buffer"() -> (w557:T17)
            n379 = property on="Lower chart" class="WFChart (strict)"("XScale.Multiplier"=w560) -> ()  [unwired: 2 in, 2 out]
            n380 = property on="Upper chart" class="WFChart (strict)"("XScale.Multiplier"=w560) -> ()  [unwired: 2 in, 2 out]
            n381 = flat-sequence {
              tunnel: w575 -> [w604]
              tunnel: [w603] -> w571
              tunnel: w573 -> [_]
              frame #0 {
                n382 = local write "Upper chart"(w604) -> ()
                n383 = local read "Zoom time X"() -> (w603:bool)
              }
            }
            n384 = call-dynamic "InitFFT_Buffer.vi"("FFT buffer size"="FFT buffer size", "dimension size"=w561, "Transfer speed"="Transfer speed", "ScopeBase In"=w566) -> ("ScopeBase Out"=w565:refnum<class "Scope5782_six_channel.lvclass">)  [unwired: 6 in, 1 out]
            n385 = local read "Show buffers"() -> (w555:bool)
            n386 = local read "Display"() -> (w556:T18)
            n387 = call "UpdateGraphs.vi"("Transfer speed"="Transfer speed", "Show buffers"=w555, "Buffer mode"=w557, "Display mode"=w556, "Graph_refs"=w559) -> ()  [unwired: 6 in, 1 out]
            n388 = property on="Zoom time X" class="Bool (strict)"("Val(Sgnl)"=w571) -> ()  [unwired: 2 in, 2 out]
          }
          event "Samples per 5782 record": Value Change {
            n389 = event-data() -> ()  [unwired: 1 in, 6 out]
            n390 = call-dynamic "SetRecordLength.vi"("Samples per 5782 record"="Samples per 5782 record", "ScopeBase In"=w608) -> ("ScopeBase Out"=w606:refnum<class "Scope5782_six_channel.lvclass">)  [unwired: 8 in, 1 out]
          }
          event "Singleshot": Value Change {
            n391 = event-data() -> ()  [unwired: 1 in, 6 out]
            n392 = local write "Rumode"(FALSE ("Rumode")) -> ()
            n393 = call-dynamic "SetRunMode.vi"("RunMode"=ScopeMode."Single" ("scope mode"), "ScopeBase in"=w610) -> ("ScopeBase out"=w611:refnum<class "Scope5782_six_channel.lvclass">)  [unwired: 8 in, 1 out]
          }
          event "Rumode": Value Change {
            n394 = event-data() -> ()  [unwired: 1 in, 6 out]
            n395 = case shown="\"Triggered\"" "Trigmode" {
              tunnel: [ScopeMode."Running" ("scope mode") ScopeMode."Continuous" ("scope mode")] -> w618
              frame "Triggered" {
              }
              frame "Continuous" {
              }
            }
            n396 = Select(t=w618, s="Rumode", f=ScopeMode."Stopped" ("scope mode")) -> (s? t:f=w617:T29)
            n397 = call-dynamic "SetRunMode.vi"("RunMode"=w617, "ScopeBase in"=w616) -> ("ScopeBase out"=w614:refnum<class "Scope5782_six_channel.lvclass">)  [unwired: 8 in, 1 out]
          }
          event "Unwrap phase": Value Change {
            w625 = dbl[][] [] ("History Data")
            n398 = event-data() -> ()  [unwired: 1 in, 6 out]
            n399 = property on="Lower chart" class="WFChart (strict)"("History Data"=w625) -> ()  [unwired: 2 in, 2 out]
            n400 = property on="Upper chart" class="WFChart (strict)"("History Data"=w625) -> ()  [unwired: 2 in, 2 out]
          }
          event "stop": Value Change {
            n401 = event-data() -> ()  [unwired: 1 in, 6 out]
          }
          event Value Change {
            n402 = event-data() -> ()  [unwired: 1 in, 6 out]
            n403 = case shown="\"V\"" "Unit" {
              tunnel: ["V" "dBV" "V^2"] -> w633
              frame "V" {
              }
              frame "dBV" {
              }
              frame "V^2" {
              }
            }
            n404 = Concatenate Strings("Amplitude [", w633, "]") -> (w631:string)
            n405 = property on="freqdata" class="WFGraph (strict)"("YScale.NameLbl.Text"=w631) -> ()  [unwired: 2 in, 2 out]
          }
          event "#bins": Value Change {
            n406 = event-data() -> ()  [unwired: 1 in, 6 out]
            n407 = local read "Upper chart"() -> (w644:dbl[][])
            n408 = local read "Window"() -> (w645:T13)
            n409 = local read "Unit"() -> (w646:T12)
            n410 = call "calc FFT_indexed.vi"("#bins"="#bins", "IQ indexes"=i32[][] [[0, 1], [2, 3], [4, 5], [6, 7], [8, 9], [10, 11], [12, 13]], "dt"=1e-06, "Unit"=w646, "Window"=w645, "data"=w644) -> ("Power Spectrum / PSD"=w643:cluster{"f0":dbl, "df":dbl, "magnitude":dbl[]}[])  [unwired: 4 in, 1 out]
            n411 = local write "freqdata"(w643) -> ()
          }
          event "Zoom time X", "Zoom time Y": Value Change {
            n412 = event-data() -> ()  [unwired: 1 in, 6 out]
            n413 = control-ref of="Upper chart"() -> (w652:refnum<vi>)
            n414 = control-ref of="Upper graph"() -> (w653:refnum<vi>)
            n415 = call "setZoomTool.vi"("Zoom Y"="Zoom time Y", "Zoom  X"="Zoom time X", "reference"=w652) -> ()  [unwired: 9 in]
            n416 = call "setZoomTool.vi"("Zoom Y"="Zoom time Y", "Zoom  X"="Zoom time X", "reference"=w653) -> ()  [unwired: 9 in]
          }
          event "Zoom freq Y", "Zoom freq X": Value Change {
            n417 = event-data() -> ()  [unwired: 1 in, 6 out]
            n418 = control-ref of="Lower chart"() -> (w660:refnum<vi>)
            n419 = control-ref of="Lower graph"() -> (w659:refnum<vi>)
            n420 = control-ref of="Adaptive FF graph"() -> (w656:refnum<vi>)
            n421 = control-ref of="freqdata"() -> (w661:refnum<vi>)
            n422 = call "setZoomTool.vi"("Zoom Y"="Zoom freq Y", "Zoom  X"="Zoom freq X", "reference"=w661) -> ()  [unwired: 9 in]
            n423 = call "setZoomTool.vi"("Zoom Y"="Zoom freq Y", "Zoom  X"="Zoom freq X", "reference"=w656) -> ()  [unwired: 9 in]
            n424 = call "setZoomTool.vi"("Zoom Y"="Zoom freq Y", "Zoom  X"="Zoom freq X", "reference"=w660) -> ()  [unwired: 9 in]
            n425 = call "setZoomTool.vi"("Zoom Y"="Zoom freq Y", "Zoom  X"="Zoom freq X", "reference"=w659) -> ()  [unwired: 9 in]
          }
          event "Show buffers": Value Change {
            n426 = event-data() -> ("CtlRef"=w669:refnum<vi>)  [unwired: 1 in, 5 out]
            n427 = control-ref of="Show buffers"() -> (w668:refnum<vi>)
            n428 = Equal?(x=w669, y=w668) -> (x = y?=w667:bool)
            n429 = case shown="False" w667 {
              frame False {
                w675 = dbl[][] [] ("History Data")
                n430 = local write "freqdata"(cluster{"f0":dbl, "df":dbl, "magnitude":dbl[]}[] [] ("freqdata")) -> ()
                n431 = property on="Upper chart" class="WFChart (strict)"("History Data"=w675) -> ()  [unwired: 2 in, 2 out]
                n432 = local write "Lower graph"(w675) -> ()
                n433 = property on="Lower chart" class="WFChart (strict)"("History Data"=w675) -> ()  [unwired: 2 in, 2 out]
                n434 = local write "Upper graph"(w675) -> ()
              }
              frame True {
              }
            }
            n435 = local read "Transfer speed"() -> (w663:T2)
            n436 = call "UpdateGraphs.vi"("Transfer speed"=w663, "Show buffers"="Show buffers", "Buffer mode"="Buffer", "Display mode"="Display", "Graph_refs"=w672) -> ("Graph_refs out"=w665:T15)  [unwired: 6 in]
            n437 = call "UpdateGraphLegends.vi"("Display"="Display", "Graph_refs"=w665) -> ()  [unwired: 9 in, 1 out]
            n438 = property on="Zoom time X" class="Bool (strict)"("Val(Sgnl)"=TRUE ("Value (Signaling)")) -> ()  [unwired: 2 in, 2 out]
          }
          event "Feed forward": Value Change {
            n439 = event-data() -> ()  [unwired: 1 in, 6 out]
            n440 = control-ref of="show feedforward"() -> (w684:refnum<vi>)
            n441 = call "LoadFeedforward.vi"("show ref"=w684, "Path"="Feed forward") -> ("error out"=w679:errorcluster, "values Q"=w680:dbl[], "values I"=w681:dbl[])  [unwired: 7 in]
            n442 = call "SetFeedForward.vi"("error in (no error)"=w679, "values Q"=w680, "values I"=w681, "Scope5785_six_channel"=w682) -> ("Scope5785_six_channel out"=w678:refnum<class "Scope5782_six_channel.lvclass">)  [unwired: 6 in, 1 out]
          }
          event "Setpoint": Value Change {
            n443 = event-data() -> ()  [unwired: 1 in, 6 out]
            n444 = control-ref of="show setpoint"() -> (w692:refnum<vi>)
            n445 = call "LoadFeedforward.vi"("show ref"=w692, "Path"="Setpoint") -> ("error out"=w687:errorcluster, "values Q"=w689:dbl[], "values I"=w690:dbl[])  [unwired: 7 in]
            n446 = call "SetSetpoint.vi"("error in (no error)"=w687, "values Q"=w689, "values I"=w690, "Scope5785_six_channel"=w688) -> ("Scope5785_six_channel out"=w686:refnum<class "Scope5782_six_channel.lvclass">)  [unwired: 6 in, 1 out]
          }
          event "Input delay 5761": Value Change {
            n447 = event-data() -> ()  [unwired: 1 in, 6 out]
            n448 = call "Read FpgaRef5761.vi"("Scope5785_six_channel"=w698) -> ("FpgaRef5761.lvclass"=w696:refnum<class "FpgaRef5761.lvclass">, "Scope5785_six_channel Out"=w697:refnum<class "Scope5782_six_channel.lvclass">)  [unwired: 8 in, 1 out]
            n449 = call "WriteSetting 32bit.vi"("value"="Input delay 5761", "FPGA Setting"=fpga_settings."Input delay", "FpgaRefBase in"=w696) -> ()  [unwired: 7 in, 2 out]
          }
          event "Count to skip 5761, stage 1", "Count to skip 5761, stage 3", "Count to skip 5761, stage 2": Value Change {
            n450 = event-data() -> ()  [unwired: 1 in, 6 out]
            n451 = call "Read FpgaRef5761.vi"("Scope5785_six_channel"=w710) -> ("FpgaRef5761.lvclass"=w708:refnum<class "FpgaRef5761.lvclass">, "Scope5785_six_channel Out"=w709:refnum<class "Scope5782_six_channel.lvclass">)  [unwired: 8 in, 1 out]
            n452 = call "WriteSetting 32bit.vi"("value"="Count to skip 5761, stage 1", "FPGA Setting"=fpga_settings."Samples to skip", "FpgaRefBase in"=w708) -> ("FpgaRefBase out"=w699:refnum<class "FpgaRef5761.lvclass">)  [unwired: 7 in, 1 out]
            n453 = call "WriteSetting 32bit.vi"("value"="Count to skip 5761, stage 2", "FPGA Setting"=fpga_settings."Samples to skip 2", "FpgaRefBase in"=w699) -> ("FpgaRefBase out"=w704:refnum<class "FpgaRef5761.lvclass">)  [unwired: 7 in, 1 out]
            n454 = call "WriteSetting 32bit.vi"("value"="Count to skip 5761, stage 3", "FPGA Setting"=fpga_settings."Samples to skip 3", "FpgaRefBase in"=w704) -> ()  [unwired: 7 in, 2 out]
          }
          event "Input delay 5782": Value Change {
            n455 = event-data() -> ()  [unwired: 1 in, 6 out]
            n456 = call "Read FpgaRef5782.vi"("Scope5785_six_channel"=w716) -> ("FpgaRef5782.lvclass"=w714:refnum<class "FpgaRef5782.lvclass">, "Scope5785_six_channel Out"=w715:refnum<class "Scope5782_six_channel.lvclass">)  [unwired: 8 in, 1 out]
            n457 = call "WriteSetting 32bit.vi"("value"="Input delay 5782", "FPGA Setting"=fpga_settings."Input delay", "FpgaRefBase in"=w714) -> ()  [unwired: 7 in, 2 out]
          }
          event "Count to skip 5782, stage 1", "Count to skip 5782, stage 2", "Count to skip 5782, stage 3": Value Change {
            n458 = event-data() -> ()  [unwired: 1 in, 6 out]
            n459 = call "Read FpgaRef5782.vi"("Scope5785_six_channel"=w728) -> ("FpgaRef5782.lvclass"=w726:refnum<class "FpgaRef5782.lvclass">, "Scope5785_six_channel Out"=w727:refnum<class "Scope5782_six_channel.lvclass">)  [unwired: 8 in, 1 out]
            n460 = call "WriteSetting 32bit.vi"("value"="Count to skip 5782, stage 1", "FPGA Setting"=fpga_settings."Samples to skip", "FpgaRefBase in"=w726) -> ("FpgaRefBase out"=w718:refnum<class "FpgaRef5782.lvclass">)  [unwired: 7 in, 1 out]
            n461 = call "WriteSetting 32bit.vi"("value"="Count to skip 5782, stage 2", "FPGA Setting"=fpga_settings."Samples to skip 2", "FpgaRefBase in"=w718) -> ("FpgaRefBase out"=w719:refnum<class "FpgaRef5782.lvclass">)  [unwired: 7 in, 1 out]
            n462 = call "WriteSetting 32bit.vi"("value"="Count to skip 5782, stage 3", "FPGA Setting"=fpga_settings."Samples to skip 3", "FpgaRefBase in"=w719) -> ()  [unwired: 7 in, 2 out]
          }
          event Value Change {
            n463 = event-data() -> ()  [unwired: 1 in, 6 out]
            n464 = call "Read FpgaRef5782.vi"("Scope5785_six_channel"=w734) -> ("FpgaRef5782.lvclass"=w732:refnum<class "FpgaRef5782.lvclass">, "Scope5785_six_channel Out"=w733:refnum<class "Scope5782_six_channel.lvclass">)  [unwired: 8 in, 1 out]
            n465 = call "WriteSetting 16bit.vi"("value"="Output scale", "FPGA Setting"=fpga_settings."Output scale", "FpgaRefBase in"=w732) -> ()  [unwired: 7 in, 2 out]
          }
          event Value Change {
            n466 = event-data() -> ()  [unwired: 1 in, 6 out]
            n467 = call "Read FpgaRef5782.vi"("Scope5785_six_channel"=w740) -> ("FpgaRef5782.lvclass"=w738:refnum<class "FpgaRef5782.lvclass">, "Scope5785_six_channel Out"=w739:refnum<class "Scope5782_six_channel.lvclass">)  [unwired: 8 in, 1 out]
            n468 = call "WriteSetting 16bit.vi"("value"="Input scale", "FPGA Setting"=fpga_settings."Input scale", "FpgaRefBase in"=w738) -> ()  [unwired: 7 in, 2 out]
          }
          event Value Change {
            n469 = event-data() -> ()  [unwired: 1 in, 6 out]
            n470 = call "Read FpgaRef5761.vi"("Scope5785_six_channel"=w744) -> ("FpgaRef5761.lvclass"=w742:refnum<class "FpgaRef5761.lvclass">, "Scope5785_six_channel Out"=w743:refnum<class "Scope5782_six_channel.lvclass">)  [unwired: 8 in, 1 out]
            n471 = call "WriteSetting 16bit.vi"("value"="Input scale 5761", "FPGA Setting"=fpga_settings."Input scale", "FpgaRefBase in"=w742) -> ()  [unwired: 7 in, 2 out]
          }
          event Value Change {
            n472 = event-data() -> ()  [unwired: 1 in, 6 out]
            n473 = call "Read FpgaRef5761.vi"("Scope5785_six_channel"=w751) -> ("FpgaRef5761.lvclass"=w749:refnum<class "FpgaRef5761.lvclass">, "Scope5785_six_channel Out"=w750:refnum<class "Scope5782_six_channel.lvclass">)  [unwired: 8 in, 1 out]
            n474 = call "WriteSetting 16bit.vi"("value"="Host scale 5761", "FPGA Setting"=fpga_settings."Host scale", "FpgaRefBase in"=w749) -> ()  [unwired: 7 in, 2 out]
          }
          event Value Change {
            n475 = event-data() -> ()  [unwired: 1 in, 6 out]
            n476 = call "Read FpgaRef5782.vi"("Scope5785_six_channel"=w758) -> ("FpgaRef5782.lvclass"=w756:refnum<class "FpgaRef5782.lvclass">, "Scope5785_six_channel Out"=w757:refnum<class "Scope5782_six_channel.lvclass">)  [unwired: 8 in, 1 out]
            n477 = call "WriteSetting 16bit.vi"("value"="Host scale", "FPGA Setting"=fpga_settings."Host scale", "FpgaRefBase in"=w756) -> ()  [unwired: 7 in, 2 out]
          }
          event "dw LP filter cut off frequency": Value Change {
            n478 = event-data() -> ()  [unwired: 1 in, 6 out]
            n479 = call "Read FpgaRef5761.vi"("Scope5785_six_channel"=w760) -> ("FpgaRef5761.lvclass"=w762:refnum<class "FpgaRef5761.lvclass">, "Scope5785_six_channel Out"=w759:refnum<class "Scope5782_six_channel.lvclass">)  [unwired: 8 in, 1 out]
            n480 = call "Write dw LP IIR coeffs.vi"("Fs [MHz}"=10.0, "cutoff fequency [MHz]"="dw LP filter cut off frequency", "FpgaRef5761"=w762) -> ()  [unwired: 8 in, 1 out]
          }
          event "Vi Vq LP  filter cutoff fequency": Value Change {
            n481 = event-data() -> ()  [unwired: 1 in, 6 out]
            n482 = call "Read FpgaRef5761.vi"("Scope5785_six_channel"=w767) -> ("FpgaRef5761.lvclass"=w768:refnum<class "FpgaRef5761.lvclass">, "Scope5785_six_channel Out"=w766:refnum<class "Scope5782_six_channel.lvclass">)  [unwired: 8 in, 1 out]
            n483 = call "Write Vi Vq IIR LP coeffs.vi"("Fs [MHz}"=10.0, "cutoff fequency [MHz]"="Vi Vq LP  filter cutoff fequency", "FpgaRef5761"=w768) -> ()  [unwired: 8 in, 1 out]
          }
          event "Vfi Vfq LP filter cut off frequency": Value Change {
            n484 = event-data() -> ()  [unwired: 1 in, 6 out]
            n485 = call "Read FpgaRef5761.vi"("Scope5785_six_channel"=w773) -> ("FpgaRef5761.lvclass"=w774:refnum<class "FpgaRef5761.lvclass">, "Scope5785_six_channel Out"=w772:refnum<class "Scope5782_six_channel.lvclass">)  [unwired: 8 in, 1 out]
            n486 = call "Write Vfi Vfq IIR LP coeffs.vi"("Fs [MHz}"=10.0, "cutoff fequency [MHz]"="Vfi Vfq LP filter cut off frequency", "FpgaRef5761"=w774) -> ()  [unwired: 8 in, 1 out]
          }
          event "w12 LP  filter cutoff fequency": Value Change {
            n487 = event-data() -> ()  [unwired: 1 in, 6 out]
            n488 = call "Read FpgaRef5761.vi"("Scope5785_six_channel"=w779) -> ("FpgaRef5761.lvclass"=w780:refnum<class "FpgaRef5761.lvclass">, "Scope5785_six_channel Out"=w778:refnum<class "Scope5782_six_channel.lvclass">)  [unwired: 8 in, 1 out]
            n489 = call "Write w12 LP IIR coeffs.vi"("Fs [MHz}"=10.0, "cutoff fequency [MHz]"="w12 LP  filter cutoff fequency", "FpgaRef5761"=w780) -> ()  [unwired: 8 in, 1 out]
          }
          event "ch1 delay", "ch3 delay": Value Change {
            n490 = event-data() -> ()  [unwired: 1 in, 6 out]
            n491 = local read "Mixer freq [MHz]"() -> (w795:dbl)
            n492 = Multiply(x="ch1 delay", y=0.001) -> (x*y=w796:dbl)
            n493 = Multiply(x="ch3 delay", y=0.001) -> (x*y=w797:dbl)
            n494 = call "Read FpgaRef5761.vi"("Scope5785_six_channel"=w786) -> ("FpgaRef5761.lvclass"=w792:refnum<class "FpgaRef5761.lvclass">, "Scope5785_six_channel Out"=w785:refnum<class "Scope5782_six_channel.lvclass">)  [unwired: 8 in, 1 out]
            n495 = Multiply(x=w795, y=6.283185307179586) -> (x*y=w793:dbl)
            n496 = Multiply(x=w796, y=w793) -> (x*y=w787:dbl)
            n497 = Multiply(x=w793, y=w797) -> (x*y=w790:dbl)
            n498 = call "WriteSetting float.vi"("value"=w787, "FPGA Setting"=fpga_settings."Fi_start", "FpgaRefBase in"=w792) -> ("FpgaRefBase out"=w791:refnum<class "FpgaRef5761.lvclass">)  [unwired: 7 in, 1 out]
            n499 = call "WriteSetting float.vi"("value"=w790, "FPGA Setting"=fpga_settings."Fi_delta", "FpgaRefBase in"=w791) -> ()  [unwired: 7 in, 2 out]
          }
          event "Update once upper", "Update once lower": Value Change {
            n500 = event-data() -> ()  [unwired: 1 in, 6 out]
            n501 = call "Write Update once lower.vi"("Update once lower"="Update once lower", "Scope5761"=w805) -> ("Scope5761"=w804:refnum<class "Scope5782_six_channel.lvclass">)  [unwired: 8 in, 1 out]
            n502 = call "Write Update once upper.vi"("Update once upper"="Update once upper", "Scope5761"=w804) -> ("Scope5761"=w803:refnum<class "Scope5782_six_channel.lvclass">)  [unwired: 8 in, 1 out]
          }
          event "Hold plot upper", "Hold plot lower": Value Change {
            w815 = T28."Enabled" ("Disabled")
            w814 = T28."Disabled and Grayed Out" ("Disabled")
            n503 = event-data() -> ()  [unwired: 1 in, 6 out]
            n504 = call "Write Hold plot upper.vi"("Hold plot upper"="Hold plot upper", "Scope5761"=w811) -> ("Scope5761"=w810:refnum<class "Scope5782_six_channel.lvclass">)  [unwired: 8 in, 1 out]
            n505 = call "Write Hold plot lower.vi"("Hold plot lower"="Hold plot lower", "Scope5761"=w810) -> ("Scope5761"=w809:refnum<class "Scope5782_six_channel.lvclass">)  [unwired: 8 in, 1 out]
            n506 = Select(t=w815, s="Hold plot upper", f=w814) -> (s? t:f=w808:T28)
            n507 = Select(t=w815, s="Hold plot lower", f=w814) -> (s? t:f=w807:T28)
            n508 = property on="Update once lower" class="Bool (strict)"("DisabledEnum"=w807) -> ()  [unwired: 2 in, 2 out]
            n509 = property on="Update once upper" class="Bool (strict)"("DisabledEnum"=w808) -> ()  [unwired: 2 in, 2 out]
          }
          event "Tau set", "Enable", "Measure Tau at Time", "Max output set": Value Change {
            n510 = event-data() -> ()  [unwired: 1 in, 6 out]
            n511 = Boolean To (0,1)(Boolean="Enable") -> (0, 1=w836:i16)
            n512 = Divide(x="Tau set", y=fxp<+/-,32,13> 6.399999618530273) -> (x/y=w835:fxp<+/-,32,13>)
            n513 = To Word Integer(number=w836) -> (16bit integer=w837:i16)
            n514 = xnode "Reinterpret Number"("x"=w835) -> ("y"=w840:fxp<+,32,32>)
            n515 = xnode "Reinterpret Number"("x"=w837) -> ("y"=w838:fxp<+/-,16,14>)
            n516 = To Fixed-Point(fixed-point type=fxp<+,16,14> 0.0, number="Max output set") -> (fixed-point=w822:fxp<+,16,14>)
            n517 = To Unsigned Long Integer(number=w840) -> (unsigned 32bit integer=w825:u32)
            n518 = xnode "Reinterpret Number"("x"=w838) -> ("y"=w826:fxp<+,16,16>)
            n519 = call "Write Setting 32bit.vi"("value"="Measure Tau at Time", "FPGA Setting"=fpga_settings."Quench t0", "ScopeBase in"=w832) -> ("ScopeBase out"=w831:refnum<class "Scope5782_six_channel.lvclass">)  [unwired: 7 in, 1 out]
            n520 = xnode "Reinterpret Number"("x"=w822) -> ("y"=w817:fxp<+,16,16>)
            n521 = call "Write Setting 32bit.vi"("value"=w825, "FPGA Setting"=fpga_settings."Quench tau set", "ScopeBase in"=w831) -> ("ScopeBase out"=w830:refnum<class "Scope5782_six_channel.lvclass">)  [unwired: 7 in, 1 out]
            n522 = call "Write Setting 16bit.vi"("value"=w826, "FPGA Setting"=fpga_settings."Quench enabled", "ScopeBase in"=w830) -> ("ScopeBase out"=w820:refnum<class "Scope5782_six_channel.lvclass">)  [unwired: 7 in, 1 out]
            n523 = call "Write Setting 16bit.vi"("value"=w817, "FPGA Setting"=fpga_settings."Quench max output", "ScopeBase in"=w820) -> ("ScopeBase out"=w818:refnum<class "Scope5782_six_channel.lvclass">)  [unwired: 7 in, 1 out]
          }
          event "Reset Quench Warning": Value Change {
            n524 = event-data() -> ()  [unwired: 1 in, 6 out]
            n525 = Boolean To (0,1)(Boolean="Reset Quench Warning") -> (0, 1=w849:i16)
            n526 = To Word Integer(number=w849) -> (16bit integer=w848:i16)
            n527 = xnode "Reinterpret Number"("x"=w848) -> ("y"=w847:fxp<+/-,16,14>)
            n528 = xnode "Reinterpret Number"("x"=w847) -> ("y"=w843:fxp<+,16,16>)
            n529 = call "Write Setting 16bit.vi"("value"=w843, "FPGA Setting"=fpga_settings."Quench reset", "ScopeBase in"=w845) -> ("ScopeBase out"=w844:refnum<class "Scope5782_six_channel.lvclass">)  [unwired: 7 in, 1 out]
          }
          event "Calculate w12": Value Change {
            n530 = event-data() -> ()  [unwired: 1 in, 6 out]
            n531 = call "Read FpgaRef5761.vi"("Scope5785_six_channel"=w854) -> ("FpgaRef5761.lvclass"=w853:refnum<class "FpgaRef5761.lvclass">, "Scope5785_six_channel Out"=w851:refnum<class "Scope5782_six_channel.lvclass">)  [unwired: 8 in, 1 out]
            n532 = call "SetW12Enabled.vi"("w12 enabled"="Calculate w12", "FpgaRef5761 In"=w853) -> ()  [unwired: 8 in, 2 out]
          }
          event "a", "b", "Fequency [kHz]": Value Change {
            n533 = event-data() -> ()  [unwired: 1 in, 6 out]
            n534 = call "SetAmPhase.vi"("b_am"="b", "a_am"="a", "fclk (MHz)"=100.0, "Am freq [kHz]"="Fequency [kHz]", "Scope5785_six_channel"=w861) -> ("Scope5785_six_channel out"=w860:refnum<class "Scope5782_six_channel.lvclass">)  [unwired: 5 in, 1 out]
          }
          event "w12 - b", "w12 - a", "w12 - dt": Value Change {
            n535 = event-data() -> ()  [unwired: 1 in, 6 out]
            n536 = To Fixed-Point(fixed-point type=fxp<+/-,32,12> 0.0 ("x"), number="w12 - a") -> (fixed-point=w881:fxp<+/-,32,12>)
            n537 = To Fixed-Point(fixed-point type=fxp<+/-,32,14> 0.0 ("x"), number="w12 - b") -> (fixed-point=w879:fxp<+/-,32,14>)
            n538 = To Fixed-Point(fixed-point type=fxp<+/-,32,26> 0.0 ("x"), number="w12 - dt") -> (fixed-point=w871:fxp<+/-,32,26>)
            n539 = call "Read FpgaRef5761.vi"("Scope5785_six_channel"=w864) -> ("FpgaRef5761.lvclass"=w885:refnum<class "FpgaRef5761.lvclass">, "Scope5785_six_channel Out"=w863:refnum<class "Scope5782_six_channel.lvclass">)  [unwired: 8 in, 1 out]
            n540 = xnode "Reinterpret Number"("x"=w881) -> ("y"=w882:fxp<+,32,32>)
            n541 = xnode "Reinterpret Number"("x"=w879) -> ("y"=w878:fxp<+,32,32>)
            n542 = xnode "Reinterpret Number"("x"=w871) -> ("y"=w872:fxp<+,32,32>)
            n543 = To Unsigned Long Integer(number=w882) -> (unsigned 32bit integer=w880:u32)
            n544 = To Unsigned Long Integer(number=w878) -> (unsigned 32bit integer=w874:u32)
            n545 = To Unsigned Long Integer(number=w872) -> (unsigned 32bit integer=w869:u32)
            n546 = call "WriteSetting 32bit.vi"("value"=w880, "FPGA Setting"=fpga_settings."w12_a", "FpgaRefBase in"=w885) -> ("FpgaRefBase out"=w876:refnum<class "FpgaRef5761.lvclass">)  [unwired: 7 in, 1 out]
            n547 = call "WriteSetting 32bit.vi"("value"=w874, "FPGA Setting"=fpga_settings."w12_b", "FpgaRefBase in"=w876) -> ("FpgaRefBase out"=w868:refnum<class "FpgaRef5761.lvclass">)  [unwired: 7 in, 1 out]
            n548 = call "WriteSetting 32bit.vi"("value"=w869, "FPGA Setting"=fpga_settings."w12_dt", "FpgaRefBase in"=w868) -> ()  [unwired: 7 in, 2 out]
          }
          event Value Change {
            n549 = event-data() -> ()  [unwired: 1 in, 6 out]
            n550 = call "Read FpgaRef5761.vi"("Scope5785_six_channel"=w894) -> ("FpgaRef5761.lvclass"=w891:refnum<class "FpgaRef5761.lvclass">, "Scope5785_six_channel Out"=w893:refnum<class "Scope5782_six_channel.lvclass">)  [unwired: 8 in, 1 out]
            n551 = To Unsigned Long Integer(number="w12 scale") -> (unsigned 32bit integer=w892:u32)
            n552 = To Unsigned Long Integer(number="dw scale") -> (unsigned 32bit integer=w888:u32)
            n553 = call "WriteSetting 32bit.vi"("value"=w892, "FPGA Setting"=fpga_settings."w12_scale", "FpgaRefBase in"=w891) -> ("FpgaRefBase out"=w889:refnum<class "FpgaRef5761.lvclass">)  [unwired: 7 in, 1 out]
            n554 = call "WriteSetting 32bit.vi"("value"=w888, "FPGA Setting"=fpga_settings."dw_scale", "FpgaRefBase in"=w889) -> ()  [unwired: 7 in, 2 out]
          }
          event "Q0 identify": Value Change {
            n555 = event-data() -> ()  [unwired: 1 in, 6 out]
            n556 = call "Set Q0 enabled.vi"("calc Q0"="Q0 identify", "Scope5761 in"=w900) -> ("Scope5761out"=w899:refnum<class "Scope5782_six_channel.lvclass">)  [unwired: 8 in, 1 out]
          }
          event "Nforget", "sigm", "Q0 - A", "Q0 - C", "Q0 - E", "Q0 - B", "Q0 - D", "Test", "Cal": Value Change {
            n557 = event-data() -> ()  [unwired: 1 in, 6 out]
            n558 = call "Read Q0 params.vi"("Scope5761 in"=w914) -> ("Q0 params"=w912:T32, "Scope5761out"=w913:refnum<class "Scope5782_six_channel.lvclass">)  [unwired: 8 in, 1 out]
            n559 = Bundle By Name(cluster=w912, "sigm"="sigm", "Nforget"="Nforget", "Q0 - A"="Q0 - A", "Q0 - B"="Q0 - B", "Q0 - C"="Q0 - C", "Q0 - D"="Q0 - D", "Q0 - E"="Q0 - E", "Test"="Test", "Cal"="Cal") -> (w902:T32)
            n560 = call "Write Q0 params.vi"("Q0 params"=w902, "Scope5761 in"=w913) -> ("Scope5761out"=w915:refnum<class "Scope5782_six_channel.lvclass">)  [unwired: 8 in, 1 out]
          }
        }
        n561 = case shown="False" w227 {
          tunnel: w226 -> [w237 _]
          frame False {
            n562 = Generate User Event(user event=w237, event data cluster=T26 {"Automatic"=TRUE, "Save"=TRUE} ("event data")) -> ()  [unwired: 2 in, 2 out]
          }
          frame True {
          }
        }
      }
      "stop 2" <- w215
    }
    frame Error {
    }
  }
  n563 = call "Run.vi"("SettingsFile in"=w23) -> ()  [unwired: 10 in, 1 out]
  n564 = Close Reference(reference=w54) -> ()  [unwired: 1 in, 1 out]
  n565 = Unregister For Events(event registration refnum=w143) -> ()  [unwired: 1 in, 1 out]
  n566 = call-dynamic "Close.vi"("ScopeBase in"=w113) -> ("error out"=w112:errorcluster)  [unwired: 10 in]
  n567 = flat-sequence {
    tunnel: w112 -> [_]
    frame #0 {
      n568 = global write "global_stop.vi" "Stop"(TRUE ("Stop")) -> ()
    }
  }
